vi "Text control 2 v5.4_pump-specific.vi"() -> ()   [LabVIEW 2016]
panel:
  in  "Tab Control":enum32{"Main", "Other parameters"}(tab)
  out "Line running":i32
  out "Total lines":i32
  out "Path":path=path "C:/users/rlp38/09Apr2009LTtesting/test2.txt"
  out "I vs Vg":cluster{"Y data in":dbl[], "X data in":dbl[]}[](graph)
  out "Is max":dbl format="%.2e"
  out "Id max":dbl format="%.2e"
  out "Ig max":dbl format="%.2e"
  out "Imax vs time":cluster{"Y data in":dbl[], "X data in":dbl[]}[](graph)
  out "Imin vs time":cluster{"Y data in":dbl[], "X data in":dbl[]}[](graph)
  out "I vs Vd":cluster{"Y data in":dbl[], "X data in":dbl[]}[](graph)
  in  "Script":string="#-------------------------------------------------------\n# SPM pump cleaning script\n#\n# Version 0.5\n# Author: Dimitrios Simatos\n# Last updated: 2018-01-05\n#-------------------------------------------------------\n# Description\n#\n# This script is designed to run the cleaning sequence of the SPM OEM pump.\n# This script needs to be run 4 times!\n#-------------------------------------------------------\n# Changes\n#\n# Placed initialization and hard stop commands in the beginning.\n#-------------------------------------------------------\n# Important points\n#\n# Never leave any liquid in the pump to dry after the experiments. If they dry, the residue may block the valve.\n# Always run the cleaning cycle after the experiments.\n# Use clockwise rotation when going up in valve port numbers and vice versa.\n#-------------------------------------------------------\n# Things to do before running the script\n#\n# Set time units to minutes.\n# Set filenames.\n# Replace the tubing, if necessary.\n#-------------------------------------------------------\n# Port connections\n#\n# Port 1: Waste\n# Port 2: Waste\n# Port 3: Various cleaning liquids\n# Port 4: Waste\n# Port 5: Waste\n# Port 6: Waste\n#\n# Between each of the 4 runs, the settings of Port 3 will change, according to the cleaning protocol.\n# The settings for Port 3 are:\n# 1st run: 1% v/v solution of sodium hypochlorite in ultrapure water\n# 2nd run: 0.1% w/v solution of sodium dodecyl sulfate in ultrapure water\n# 3rd run: Ultrapure water\n# 4th run: Waste (in air, not immersed in liquid)\n#-------------------------------------------------------\n# Cleaning protocol for the SPM OEM pump (from the manual)\n#\n# A cleaning procedure should be performed at the end of each day or in between two different experiments.\n# An effective cleaning can be performed in the following manner:\n# • Bleach solution to kill microorganisms\n# 1. Prepare a solution of 1% chlorine bleach and deionized water\n#    NOTE: Prepare a 1% v/v solution of sodium hypochlorite in deionized water\n# 2. Prepare a reservoir and place 1 tubing in the bleach solution and 5 tubings in a waste recipient\n# 3. Pick up the bleach solution through 1 port to entirely fill the syringe\n# 4. Sequentially output the syringe content through the remaining ports and throw it to the waste\n# 5. Repeat operation at least 2 times\n# • Detergent solution to remove debris\n# 1. Prepare a solution of 0.1% detergent and deionized water\n#    NOTE: Prepare a 0.1% w/v solution of sodium dodecyl sulfate in deionized water\n# 2. Move the tubing from the bleach solution reservoir and place it into a reservoir of detergent solution\n# 3. Pick up the detergent solution through 1 port to entirely fill the syringe\n# 4. Sequentially output the detergent solution through the remaining ports into the waste recipient\n# 5. Repeat operation at least 2 times\n# • Rinsing water to prepare the pump for your next experiment\n# 1. Move the tubing from the detergent solution reservoir and place it into a reservoir of deionized water\n# 2. Pick up the rinsing solution through 1 port to entirely fill the syringe\n# 3. Sequentially output the rinse water through the remaining ports into the waste recipient\n# 4. Repeat operation at least 2 times\n# • Replace the tubing, if necessary\n#-------------------------------------------------------\n# Pumping cycles and execution time\n#\n# Execution time for a single cycle: 6 x (1 min + 10 sec) = 7 minutes\n# Total execution time: 4 x 7 = 28 minutes\n# Since the script has to run 4 times, the cleaning lasts for: 4 x 28 = 112 minutes\n# Air must be the last to be pumped through the valve, to remove all liquids.\n# There are 4 pumping cycles. Each one draws a different liquid through port 3 and pumps it sequentially through ports 1,2,4,5,6.\n# During the sequential pumping, each port receives 200 ml of liquid (20% of the total syringe volume = 600 \"plunger units\")\n# The device must be disconnected from the port during the cleaning procedure.\n# All cycles are similar, except cycle 1 has the initialization command uncommented and the first report valve command commented.\n#-------------------------------------------------------\n# Volume of liquid needed\n#\n# Volume of liquid needed per cycle: 1 ml\n# Total volume of liquid needed per script run: 4 x 1 = 4 ml\n# Since the script has to run 4 times, the first 3 with different liquids, I need:\n# 4 ml of 1% v/v solution of sodium hypochlorite in ultrapure water\n# 4 ml of 0.1% w/v solution of sodium dodecyl sulfate in ultrapure water\n# 4 ml of ultrapure water\n#-------------------------------------------------------\n# Parameters\n#\n# Syringe size: 1 ml\n# Step resolution N = 0.01 mm\n# Drawing flow V = 300 pulses/second (6000 ul/min)\n# Pumping flow V = 300 pulses/second (6000 ul/min)\n#-------------------------------------------------------\n# Pump initialization\npump /1T #hard stop pump\npump /1ZR #initialize pump\n#-------------------------------------------------------\n# Cycle 1\n# Fill the syringe\npump /1Q #query pump\npump /1? #report absolute plunger position\n#pump /1?6 #report valve position\nwait-min 1 #wait 1 minute\npump /1N0R #set step resolution: 0.01 mm\npump /1Q #query pump\npump /1? #report absolute plunger position (the plunger should be at 0)\npump /1?6 #report valve position\nwait 1000 #wait 1 second\npump /1V300R #choose speed: 300 steps/s (6000 ul/min)\npump /1Q #query pump\nwait 1000 #wait 1 second\npump /1I3R #go to port 3, clockwise rotation\npump /1Q #query pump\npump /1?6 #report valve position\nwait 1000 #wait 1 second\npump /1A3000R #go to absolute position 3000 (= draw 1 ml)\nwait 30000 #wait 30 seconds\npump /1Q #query pump\npump /1? #report absolute plunger position (the plunger should have finished moving)\n#pump /1?6 #report valve position\n# The sequential pumping begins\n# Port 1\npump /1O1R #switch to port 1, counterclockwise rotation\npump /1Q #query pump\npump /1?6 #report valve position\npump /1A2400R #go to absolute position 2400 (= pump 200 ul)\npump /1Q #query pump\npump /1? #report absolute plunger position (the plunger should be moving to 0)\nwait-min 1 #wait 1 minute\npump /1? #report absolute plunger position (the plunger should have finished moving)\n# Port 2\npump /1I2R #switch to port 2, clockwise rotation\npump /1Q #query pump\npump /1?6 #report valve position\npump /1A1800R #go to absolute position 1800 (= pump 200 ul)\npump /1Q #query pump\npump /1? #report absolute plunger position (the plunger should be moving to 0)\nwait-min 1 #wait 1 minute\npump /1? #report absolute plunger position (the plunger should have finished moving)\n# Port 4\npump /1I4R #switch to port 4, clockwise rotation\npump /1Q #query pump\npump /1?6 #report valve position\npump /1A1200R #go to absolute position 1200 (= pump 200 ul)\npump /1Q #query pump\npump /1? #report absolute plunger position (the plunger should be moving to 0)\nwait-min 1 #wait 1 minute\npump /1? #report absolute plunger position (the plunger should have finished moving)\n# Port 5\npump /1I5R #switch to port 5, clockwise rotation\npump /1Q #query pump\npump /1?6 #report valve position\npump /1A600R #go to absolute position 600 (= pump 200 ul)\npump /1Q #query pump\npump /1? #report absolute plunger position (the plunger should be moving to 0)\nwait-min 1 #wait 1 minute\npump /1? #report absolute plunger position (the plunger should have finished moving)\n# Port 6\npump /1I6R #switch to port 6, clockwise rotation\npump /1Q #query pump\npump /1?6 #report valve position\npump /1A0R #go to absolute position 0 (= pump 200 ul)\npump /1Q #query pump\npump /1? #report absolute plunger position (the plunger should be moving to 0)\nwait-min 1 #wait 1 minute\npump /1? #report absolute plunger position (the plunger should have finished moving)\n#-------------------------------------------------------\n# Cycle 2\n# Fill the syringe\n#pump /1ZR #initialize pump\npump /1Q #query pump\npump /1? #report absolute plunger position\npump /1?6 #report valve position\nwait-min 1 #wait 1 minute\npump /1N0R #set step resolution: 0.01 mm\npump /1Q #query pump\npump /1? #report absolute plunger position (the plunger should be at 0)\npump /1?6 #report valve position\nwait 1000 #wait 1 second\npump /1V300R #choose speed: 300 steps/s (6000 ul/min)\npump /1Q #query pump\nwait 1000 #wait 1 second\npump /1O3R #go to port 3, counterclockwise rotation\npump /1Q #query pump\npump /1?6 #report valve position\nwait 1000 #wait 1 second\npump /1A3000R #go to absolute position 3000 (= draw 1 ml)\nwait 30000 #wait 30 seconds\npump /1Q #query pump\npump /1? #report absolute plunger position (the plunger should have finished moving)\n#pump /1?6 #report valve position\n# The sequential pumping begins\n# Port 1\npump /1O1R #switch to port 1, counterclockwise rotation\npump /1Q #query pump\npump /1?6 #report valve position\npump /1A2400R #go to absolute position 2400 (= pump 200 ul)\npump /1Q #query pump\npump /1? #report absolute plunger position (the plunger should be moving to 0)\nwait-min 1 #wait 1 minute\npump /1? #report absolute plunger position (the plunger should have finished moving)\n# Port 2\npump /1I2R #switch to port 2, clockwise rotation\npump /1Q #query pump\npump /1?6 #report valve position\npump /1A1800R #go to absolute position 1800 (= pump 200 ul)\npump /1Q #query pump\npump /1? #report absolute plunger position (the plunger should be moving to 0)\nwait-min 1 #wait 1 minute\npump /1? #report absolute plunger position (the plunger should have finished moving)\n# Port 4\npump /1I4R #switch to port 4, clockwise rotation\npump /1Q #query pump\npump /1?6 #report valve position\npump /1A1200R #go to absolute position 1200 (= pump 200 ul)\npump /1Q #query pump\npump /1? #report absolute plunger position (the plunger should be moving to 0)\nwait-min 1 #wait 1 minute\npump /1? #report absolute plunger position (the plunger should have finished moving)\n# Port 5\npump /1I5R #switch to port 5, clockwise rotation\npump /1Q #query pump\npump /1?6 #report valve position\npump /1A600R #go to absolute position 600 (= pump 200 ul)\npump /1Q #query pump\npump /1? #report absolute plunger position (the plunger should be moving to 0)\nwait-min 1 #wait 1 minute\npump /1? #report absolute plunger position (the plunger should have finished moving)\n# Port 6\npump /1I6R #switch to port 6, clockwise rotation\npump /1Q #query pump\npump /1?6 #report valve position\npump /1A0R #go to absolute position 0 (= pump 200 ul)\npump /1Q #query pump\npump /1? #report absolute plunger position (the plunger should be moving to 0)\nwait-min 1 #wait 1 minute\npump /1? #report absolute plunger position (the plunger should have finished moving)\n#-------------------------------------------------------\n# Cycle 3\n# Fill the syringe\n#pump /1ZR #initialize pump\npump /1Q #query pump\npump /1? #report absolute plunger position\npump /1?6 #report valve position\nwait-min 1 #wait 1 minute\npump /1N0R #set step resolution: 0.01 mm\npump /1Q #query pump\npump /1? #report absolute plunger position (the plunger should be at 0)\npump /1?6 #report valve position\nwait 1000 #wait 1 second\npump /1V300R #choose speed: 300 steps/s (6000 ul/min)\npump /1Q #query pump\nwait 1000 #wait 1 second\npump /1O3R #go to port 3, counterclockwise rotation\npump /1Q #query pump\npump /1?6 #report valve position\nwait 1000 #wait 1 second\npump /1A3000R #go to absolute position 3000 (= draw 1 ml)\nwait 30000 #wait 30 seconds\npump /1Q #query pump\npump /1? #report absolute plunger position (the plunger should have finished moving)\n#pump /1?6 #report valve position\n# The sequential pumping begins\n# Port 1\npump /1O1R #switch to port 1, counterclockwise rotation\npump /1Q #query pump\npump /1?6 #report valve position\npump /1A2400R #go to absolute position 2400 (= pump 200 ul)\npump /1Q #query pump\npump /1? #report absolute plunger position (the plunger should be moving to 0)\nwait-min 1 #wait 1 minute\npump /1? #report absolute plunger position (the plunger should have finished moving)\n# Port 2\npump /1I2R #switch to port 2, clockwise rotation\npump /1Q #query pump\npump /1?6 #report valve position\npump /1A1800R #go to absolute position 1800 (= pump 200 ul)\npump /1Q #query pump\npump /1? #report absolute plunger position (the plunger should be moving to 0)\nwait-min 1 #wait 1 minute\npump /1? #report absolute plunger position (the plunger should have finished moving)\n# Port 4\npump /1I4R #switch to port 4, clockwise rotation\npump /1Q #query pump\npump /1?6 #report valve position\npump /1A1200R #go to absolute position 1200 (= pump 200 ul)\npump /1Q #query pump\npump /1? #report absolute plunger position (the plunger should be moving to 0)\nwait-min 1 #wait 1 minute\npump /1? #report absolute plunger position (the plunger should have finished moving)\n# Port 5\npump /1I5R #switch to port 5, clockwise rotation\npump /1Q #query pump\npump /1?6 #report valve position\npump /1A600R #go to absolute position 600 (= pump 200 ul)\npump /1Q #query pump\npump /1? #report absolute plunger position (the plunger should be moving to 0)\nwait-min 1 #wait 1 minute\npump /1? #report absolute plunger position (the plunger should have finished moving)\n# Port 6\npump /1I6R #switch to port 6, clockwise rotation\npump /1Q #query pump\npump /1?6 #report valve position\npump /1A0R #go to absolute position 0 (= pump 200 ul)\npump /1Q #query pump\npump /1? #report absolute plunger position (the plunger should be moving to 0)\nwait-min 1 #wait 1 minute\npump /1? #report absolute plunger position (the plunger should have finished moving)\n#-------------------------------------------------------\n# Cycle 4\n# Fill the syringe\n#pump /1ZR #initialize pump\npump /1Q #query pump\npump /1? #report absolute plunger position\npump /1?6 #report valve position\nwait-min 1 #wait 1 minute\npump /1N0R #set step resolution: 0.01 mm\npump /1Q #query pump\npump /1? #report absolute plunger position (the plunger should be at 0)\npump /1?6 #report valve position\nwait 1000 #wait 1 second\npump /1V300R #choose speed: 300 steps/s (6000 ul/min)\npump /1Q #query pump\nwait 1000 #wait 1 second\npump /1O3R #go to port 3, counterclockwise rotation\npump /1Q #query pump\npump /1?6 #report valve position\nwait 1000 #wait 1 second\npump /1A3000R #go to absolute position 3000 (= draw 1 ml)\nwait 30000 #wait 30 seconds\npump /1Q #query pump\npump /1? #report absolute plunger position (the plunger should have finished moving)\n#pump /1?6 #report valve position\n# The sequential pumping begins\n# Port 1\npump /1O1R #switch to port 1, counterclockwise rotation\npump /1Q #query pump\npump /1?6 #report valve position\npump /1A2400R #go to absolute position 2400 (= pump 200 ul)\npump /1Q #query pump\npump /1? #report absolute plunger position (the plunger should be moving to 0)\nwait-min 1 #wait 1 minute\npump /1? #report absolute plunger position (the plunger should have finished moving)\n# Port 2\npump /1I2R #switch to port 2, clockwise rotation\npump /1Q #query pump\npump /1?6 #report valve position\npump /1A1800R #go to absolute position 1800 (= pump 200 ul)\npump /1Q #query pump\npump /1? #report absolute plunger position (the plunger should be moving to 0)\nwait-min 1 #wait 1 minute\npump /1? #report absolute plunger position (the plunger should have finished moving)\n# Port 4\npump /1I4R #switch to port 4, clockwise rotation\npump /1Q #query pump\npump /1?6 #report valve position\npump /1A1200R #go to absolute position 1200 (= pump 200 ul)\npump /1Q #query pump\npump /1? #report absolute plunger position (the plunger should be moving to 0)\nwait-min 1 #wait 1 minute\npump /1? #report absolute plunger position (the plunger should have finished moving)\n# Port 5\npump /1I5R #switch to port 5, clockwise rotation\npump /1Q #query pump\npump /1?6 #report valve position\npump /1A600R #go to absolute position 600 (= pump 200 ul)\npump /1Q #query pump\npump /1? #report absolute plunger position (the plunger should be moving to 0)\nwait-min 1 #wait 1 minute\npump /1? #report absolute plunger position (the plunger should have finished moving)\n# Port 6\npump /1I6R #switch to port 6, clockwise rotation\npump /1Q #query pump\npump /1?6 #report valve position\npump /1A0R #go to absolute position 0 (= pump 200 ul)\npump /1Q #query pump\npump /1? #report absolute plunger position (the plunger should be moving to 0)\nwait-min 1 #wait 1 minute\npump /1? #report absolute plunger position (the plunger should have finished moving)\n#-------------------------------------------------------"
  out "Command running:":string
  out "Serial port data":string
  out "Elapsed Time":dbl caption="Elapsed Time (s)"
  in  "Units":u16(ring)=1 items=["Seconds", "Minutes", "Hours"]
  in  "Time Offset":dbl caption="Set Start Time (s)"
  in  "Reset":bool
  in  "Auto Reset":bool
  in  "integration time":u32(slide) max=2 step=1 scale=0.0..2.0
  in  "Interrupt run":bool
  out "Absolute plunger position vs time":cluster{"Y data in":dbl[], "X data in":dbl[]}[](graph)
  out "Valve position vs time":cluster{"Y data in":dbl[], "X data in":dbl[]}[](graph)
  in  "Halt pump":bool
  in  "Hard stop pump":bool
  out "Is on":dbl format="%.2e"
  out "Id on":dbl format="%.2e"
  out "Ig on":dbl format="%.2e"
  out "Ion vs time":cluster{"Y data in":dbl[], "X data in":dbl[]}[](graph)
  out "Ioff vs time":cluster{"Y data in":dbl[], "X data in":dbl[]}[](graph)
  out "Ig min":dbl format="%.2e"
  out "Id min":dbl format="%.2e"
  out "Is min":dbl format="%.2e"
  out "Is off":dbl format="%.2e"
  out "Id off":dbl format="%.2e"
  out "Ig off":dbl format="%.2e"
  in  "Gate Range\nmode":u16(ring) items=["Auto", "Limited", "Fixed"]
  in  "Gate Range":u8(slide)=6 max=11 scale=0.0..11.0
  in  "Source/Drain\nRange mode":u16(ring) items=["Auto", "Limited", "Fixed"]
  in  "Source/Drain Range":u8(slide)=6 max=11 scale=0.0..11.0
  in  "Panel Controls":T1={"Emergency Stop"=refnum, "TransGraph Max"=1e-05, "Text/Graph (text=false)"=TRUE} {"TransGraph Max" format="%.2e"}
  in  "Panel Controls 2":T2={"Emergency Stop"=refnum, "TransGraph Max"=1e-05, "Text/Graph (text=false)"=TRUE, "TransGraph Min"=1e-11} {"TransGraph Min" format="%.2e"; "TransGraph Max" format="%.2e"}
  in  "SMU4":cluster{"on/off":bool, "Voltage":dbl} {"Voltage" min=-100.0 max=100.0 format="%.2f"}
  in  "Full Reset":bool
  in  "Standby":T3
  out "error out":errorcluster
  in  "Delay before read (ms)":u32=1000
  in  "byte count":u32=64
  in  "Serial End Mode for Reads":u16(ring)=2 items=["None", "LastBit", "TermChar"]
  in  "Timeout (ms)":u32=10000
  in  "Enable Termination\nChar (T)":bool=TRUE
  in  "Termination char\n(0xA = '\\n' = LF)\n(0xD = '\\r' = CR)":u8=13 format="%.0x"
  in  "flow control":u16(ring) items=["None"=0, "XON/XOFF"=1, "RTS/CTS"=2, "DTR/DSR"=4]
  in  "stop bits":u16(ring)=10 items=["1.0"=10, "1.5"=15, "2.0"=20]
  in  "parity":u16(ring) items=["None", "Odd", "Even", "Mark", "Space"]
  in  "data bits":u16=8 min=5 max=8 step=1
  in  "VISA resource name":refnum<visa-resource-name>="COM6"
  in  "baud rate":u32=9600
  in  "Drain: Compliance":dbl=0.001 format="%.8f"
  in  "Gate: Compliance":dbl=0.001 format="%.8f"
  in  "hold time /s":dbl format="%.2f"
  in  "delay time /s":dbl format="%.2f"
  in  "Integration time (short)":dbl=0.0019 min=8e-05 max=0.0019 step=8e-05 format="%^.0e"
  in  "Integration time (long)":dbl=0.32 min=0.04 max=2.0 step=0.02 format="%.2f"
  in  "Step delay /s":dbl format="%.2f"
  in  "Filename (variable part)":string="step_1_up-H2O_initial_"
  in  "Suffix (script)":string="script.txt"
  in  "Gate":T4={"Gate Start"=0.0, "Gate Stop"=2.0, "Gate Step (linear only)"=1.0, "Gate Compliance"=0.0001, "Gate PComp"=0.0, "Range mode"=0, "Range"=6} {"Range" max=11 scale=0.0..11.0; "Range mode" items=["Auto", "Limited", "Fixed"]; "Gate PComp" format="%^.2e"; "Gate Compliance" format="%^.2e"; "Gate Step (linear only)" format="%^.4e"; "Gate Stop" format="%^.4e"; "Gate Start" format="%^.4e"}
  in  "Drain 2":T5={"Drain Start"=0.0, "Drain Stop"=2.0, "Drain Compliance"=0.0001, "Drain Step"=1.0, "Drain PComp"=0.0, "Range mode"=0, "Range"=6} {"Range" max=11 scale=0.0..11.0; "Range mode" items=["Auto", "Limited", "Fixed"]; "Drain PComp" format="%^.2e"; "Drain Step" format="%^.4e"; "Drain Compliance" format="%^.2e"; "Drain Stop" format="%^.4e"; "Drain Start" format="%^.4e"}
  in  "Timings 2":T6={"integration time"=0, "Short/Long integration time"=0.00064, "hold time (sec)"=0.0, "delay time (sec)"=0.0, "Step Time (0 disables)"=0.0, "sweep method"=0, "Pulse period"=0.005, "Base voltage"=0.0, "Pulse width"=0.0005} {"Pulse width" min=0.0005 max=0.1 step=0.0001 format="%.4f"; "Base voltage" format="%^.4e"; "Pulse period" min=0.005 max=1.0 step=0.0001 format="%.4f"; "sweep method" items=["Continuous", "Pulsed"]; "Step Time (0 disables)" format="%.2f"; "delay time (sec)" format="%.4f"; "hold time (sec)" format="%.4f"; "Short/Long integration time" format="%^.0e"; "integration time" scale=0.0..2.0}
  # "Syntax:\nitime [s|m|l]\ngaterangemode [a|l|f]\ndrainrangemode [a|l|f]\npulsed [on|off] PulsePeriod(sec) PulseBaseVoltage PulseONWidth(sec)\nstandby [on l off]\nwait NumMilliseconds\nwait-min NumMinutes\n# texthere = comment\ntransfer [s|d] VgStart VgStop VgStep VdStart VdStop VdStep\noutput [s|d] VgStart VgStop VgStep VdStart VdStop VdStep\nsample Vg Vd NumSamples Time(s) SampleInterval(s)\nsamplei Idg NumSamples Time(s) SampleInterval(s) VDGcompliance\n100 samples is approximately 13 seconds with medium integration\n# if in doubt use SampleInterval(s) = 0.004\nstressV VG VD IGcompliance IDcompliance Duration(sec)\nstressI IDG VDGcompliance Duration(sec)\nvsu2pulse Bias Duration(s)\npulsedstressV [s|d] VEstop VgON VgOFF Period(s) PulseONwidth(s) Vd\nsample-fpp Vg Vd NumSamples Time\nresample-fpp Vg Vd\ntransfer-fpp [s|d] VgStart VgStop VgStep VdStart VdStop VdStep\noutput-fpp [s|d] VgStart VgStop VgStep VdStart VdStop VdStep\nserial SerialPortCommand\npump SerialPortCommand for the SPM pump\n\nSPM Pump Syntax (<x>: pump number, use 1 if only one pump):\nif the command syntax contains [R], then append the letter R to the command\n/<x>Q: query (a query command should follow each command)\n/<x>Z[R] or /<x>Y[R]: initialize pump\n/<x>N<n>[R] (<n>=0,1): <0> (<1>) microstep 0.01 mm (0.00125 mm) resolution\n/<x>I<n> (<n>=0-6): turn to port number n (clockwise)\n/<x>O<n> (<n>=0-6): turn to port number n (counterclockwise)\n/<x>X: Re-execute last command string\n/<x>G<n>[R] (<n>=0-60000): repeat command sequence (default: 0, 0=loop forever)\n/<x>g: Mark the start of a repeat sequence (max = 10)\n/<x>M<n>[R] (<n>=0-86400000): delay command execution by n milliseconds\n/<x>H: Halt; Pause the sequence after finishing the current move\n/<x>T: Hardstop; Interrupt the current move and suppress it from the sequence\n/<x>A<n>[R] (<n>=0-3000 with N=0, 0-24000 with N=1): absolute position\n/<x>P<n>[R] (<n>=0-3000 with N=0, 0-24000 with N=1): relative pickup\n/<x>D<n>[R] (<n>=0-3000 with N=0, 0-24000 with N=1): relative dispense\n/<x>V<n>[R] (<n>=1-1600 default: 150): set peak speed (pulses/sec)\nNOTE: The lowest speed limit is 1 pulse/sec, not 5, as the manual states.\n/<x>S<n>[R] (<n>=10-40 default: 22): set speed (NOT in pulses/sec, look in manual)\nNOTE: When controlled with absolute position, one does not need to pay special attention to the syringe that is mounted on the pump.\nWithdraw from lower stage (ports 3, 5), dispense from higher stage (ports 2, 4, 6).\nConnect Port 1 to waste."
  # "Time"
  # "1\n2\n3\n4\n5\n6\n7\n8\n9\n10\n11\n12\n13\n14\n15\n16\n17\n18\n19\n20"
  # "Serial port settings"
  # "Filename settings"
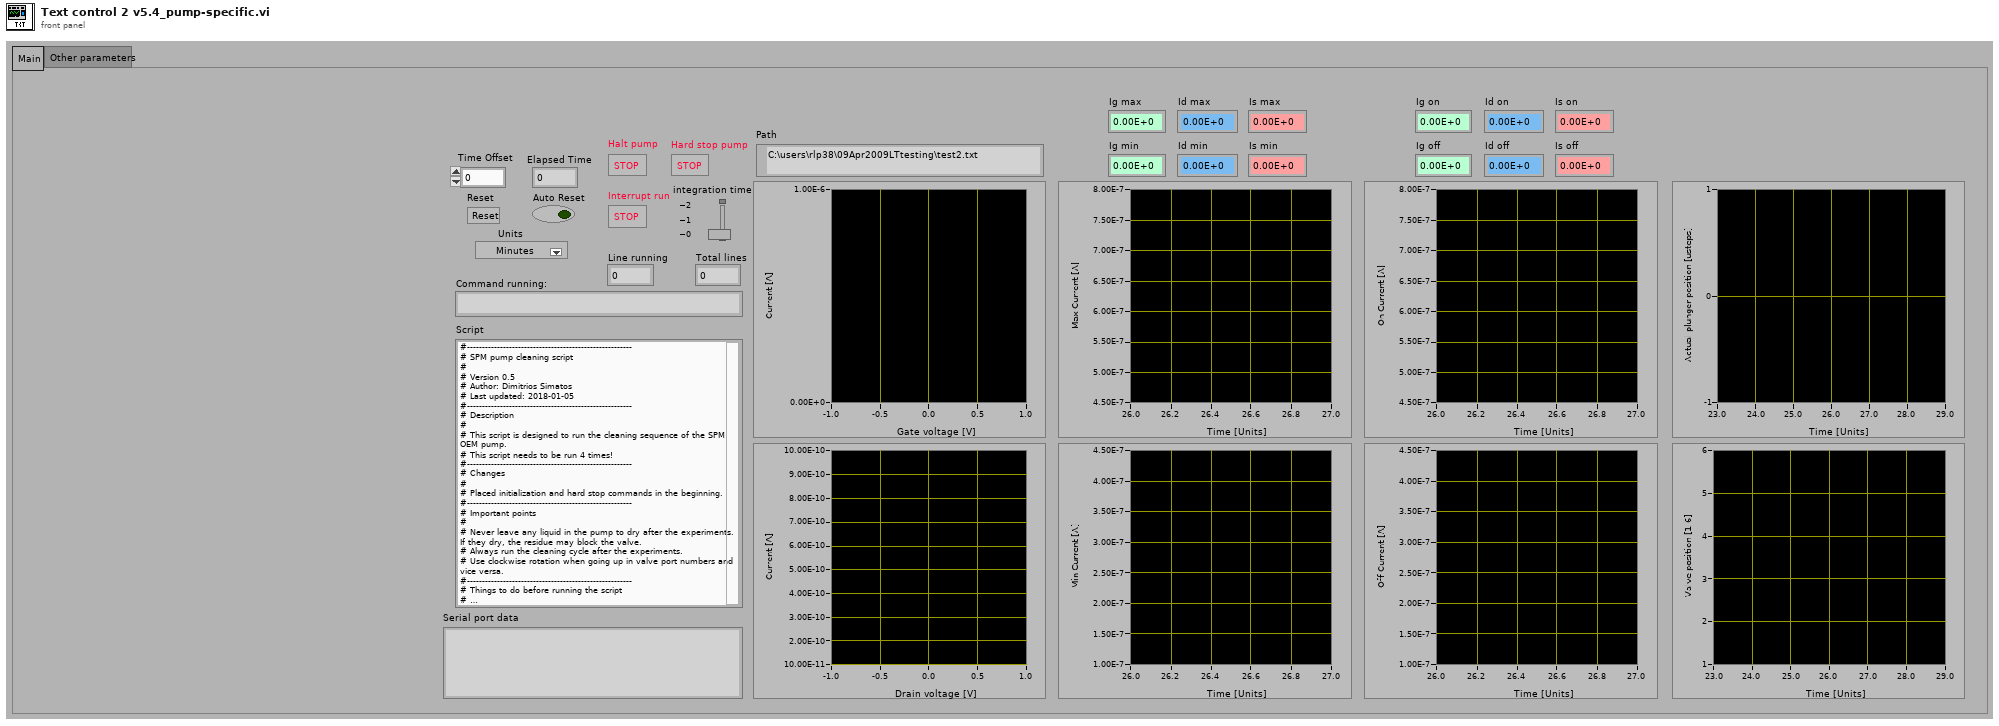
[diagram p1: front panel]
types:
  T1 = cluster{"Emergency Stop":refnum<vi>, "TransGraph Max":dbl, "Text/Graph (text=false)":bool}
  T2 = cluster{"Emergency Stop":refnum<vi>, "TransGraph Max":dbl, "Text/Graph (text=false)":bool, "TransGraph Min":dbl}
  T3 = cluster{"Gate Standby":bool, "Drain Standby":bool}
  T4 = cluster{"Gate Start":dbl, "Gate Stop":dbl, "Gate Step (linear only)":dbl, "Gate Compliance":dbl, "Gate PComp":dbl, "Range mode":u16, "Range":u8}
  T5 = cluster{"Drain Start":dbl, "Drain Stop":dbl, "Drain Compliance":dbl, "Drain Step":dbl, "Drain PComp":dbl, "Range mode":u16, "Range":u8}
  T6 = cluster{"integration time":u32, "Short/Long integration time":dbl, "hold time (sec)":dbl, "delay time (sec)":dbl, "Step Time (0 disables)":dbl, "sweep method":u16, "Pulse period":dbl, "Base voltage":dbl, "Pulse width":dbl}
  T7 = enum16{"open", "replace", "create", "open or create", "replace or create", "replace or create with confirmation"}
  T8 = cluster{"V2 Start":dbl, "V2 Step":dbl, "Number of points":i32}
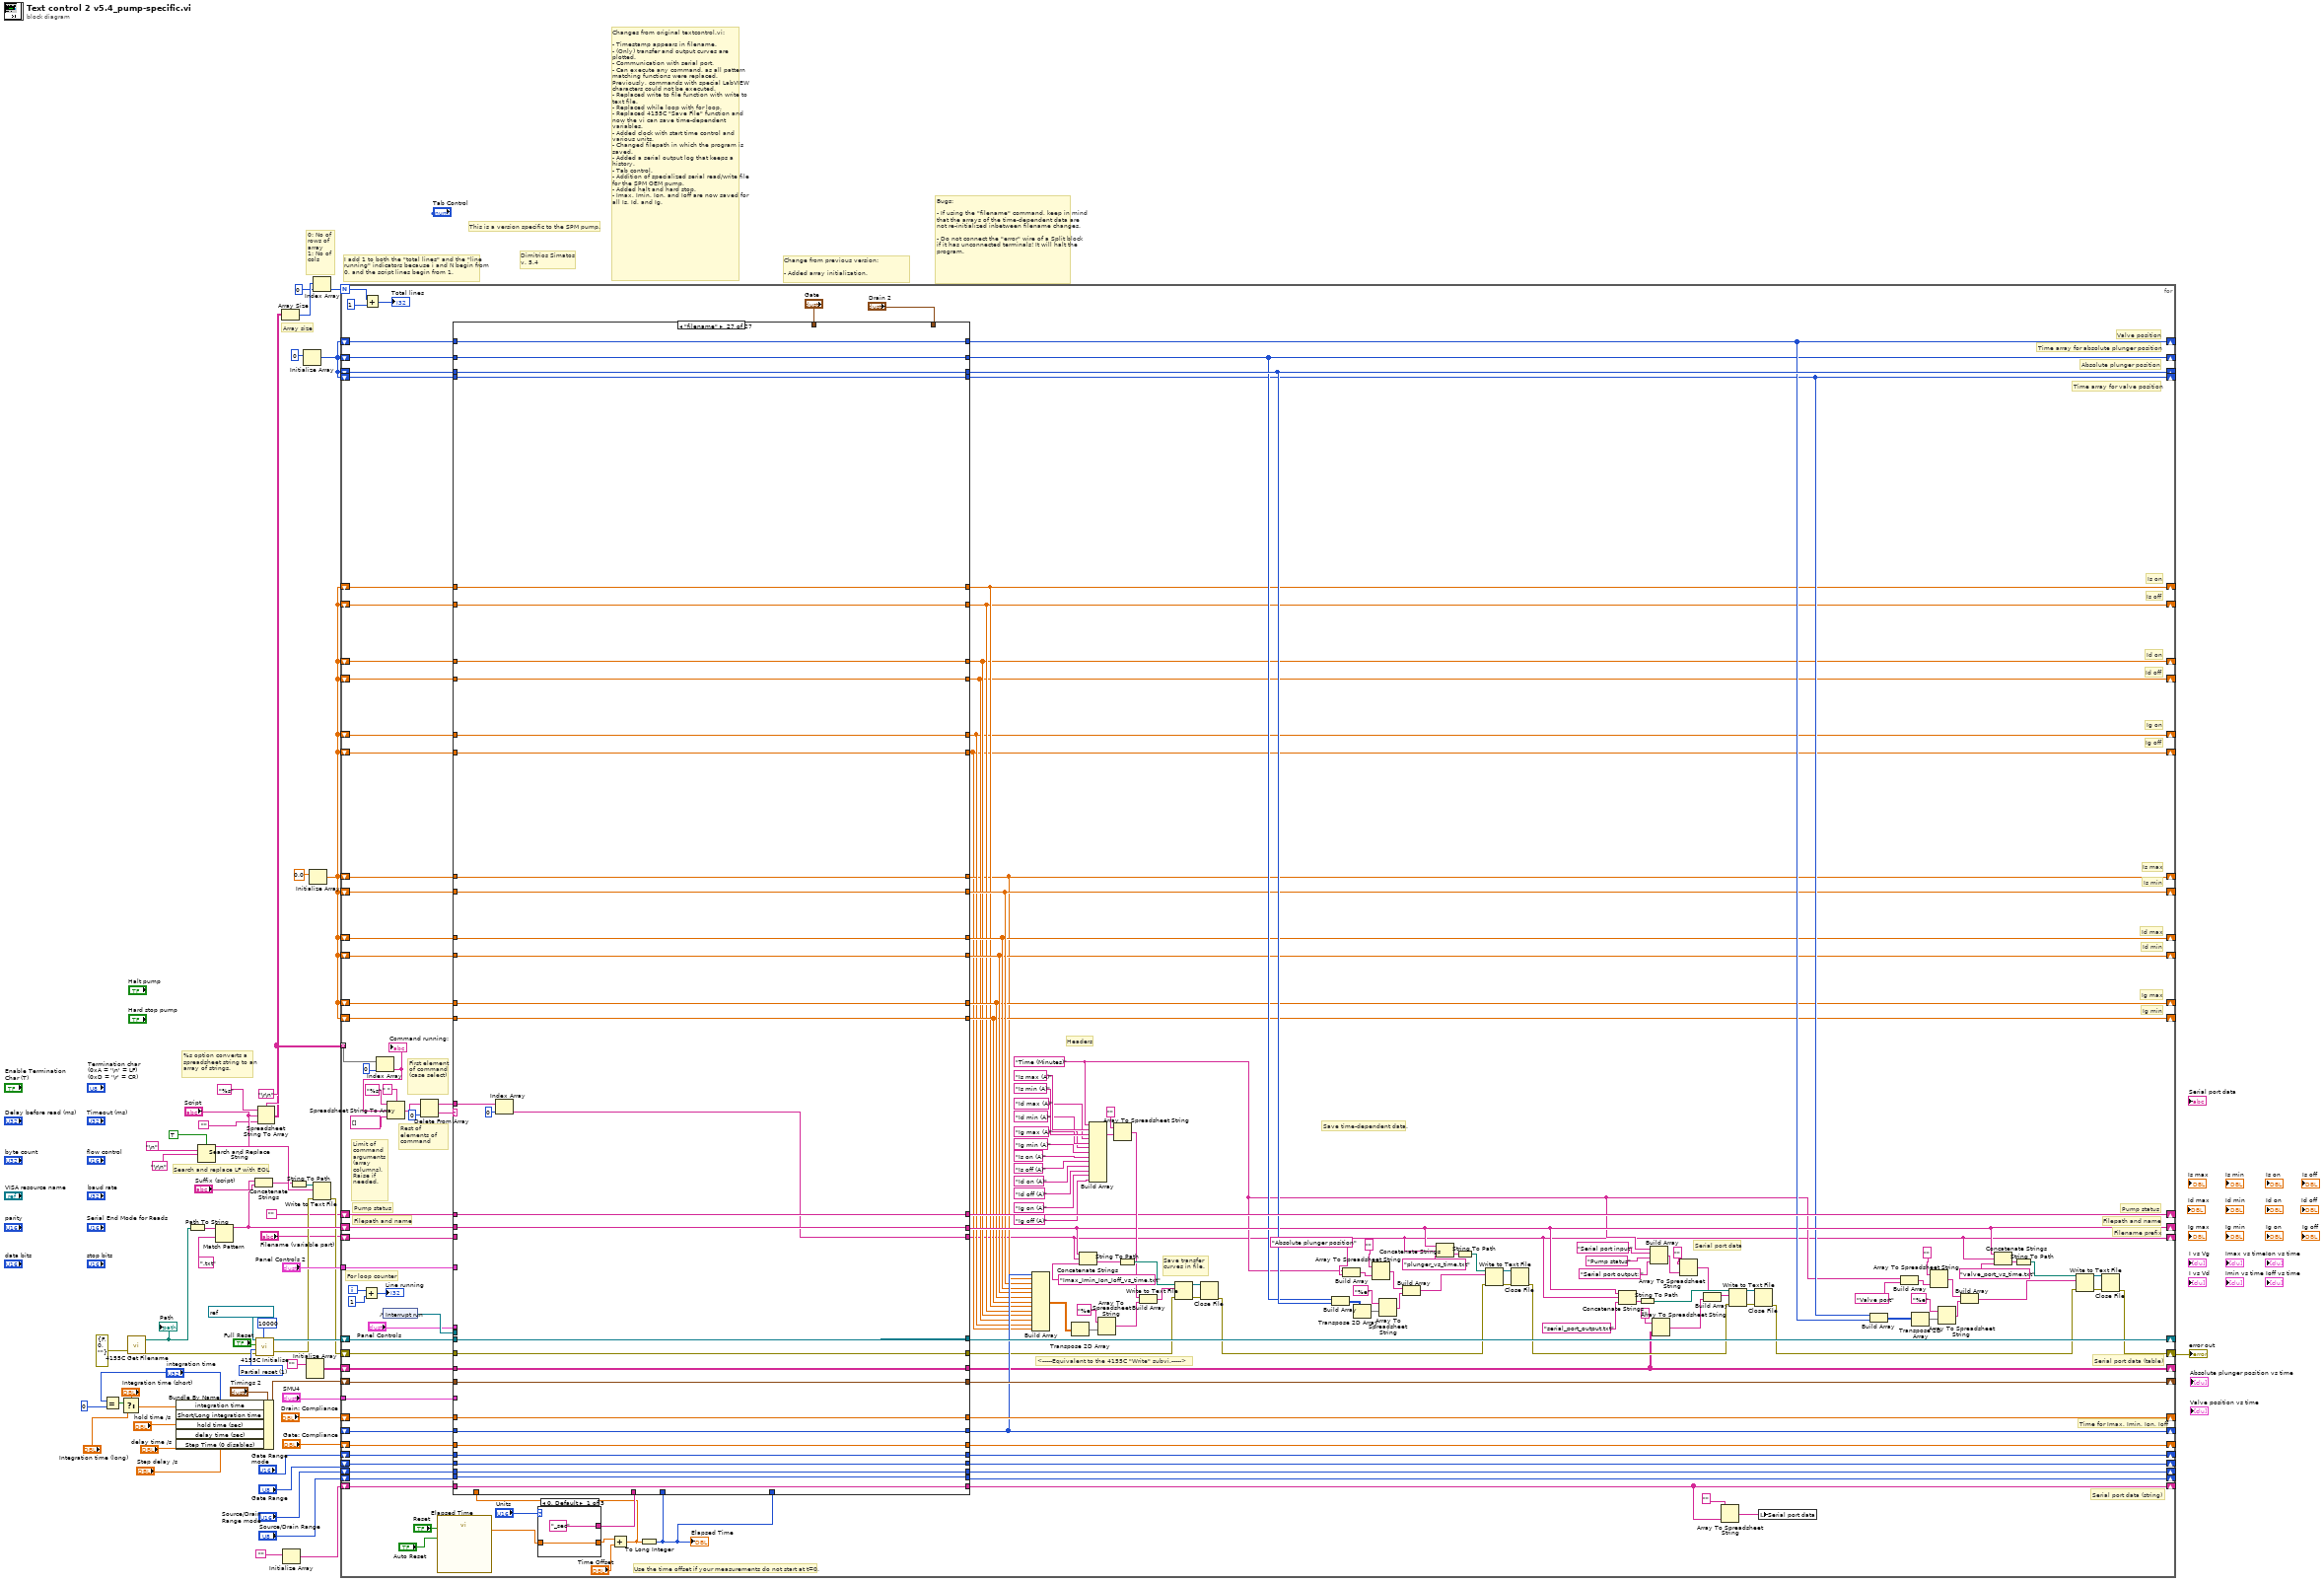
[diagram p0: block diagram]
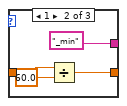
[diagram p2: hidden frame]
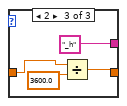
[diagram p3: hidden frame]
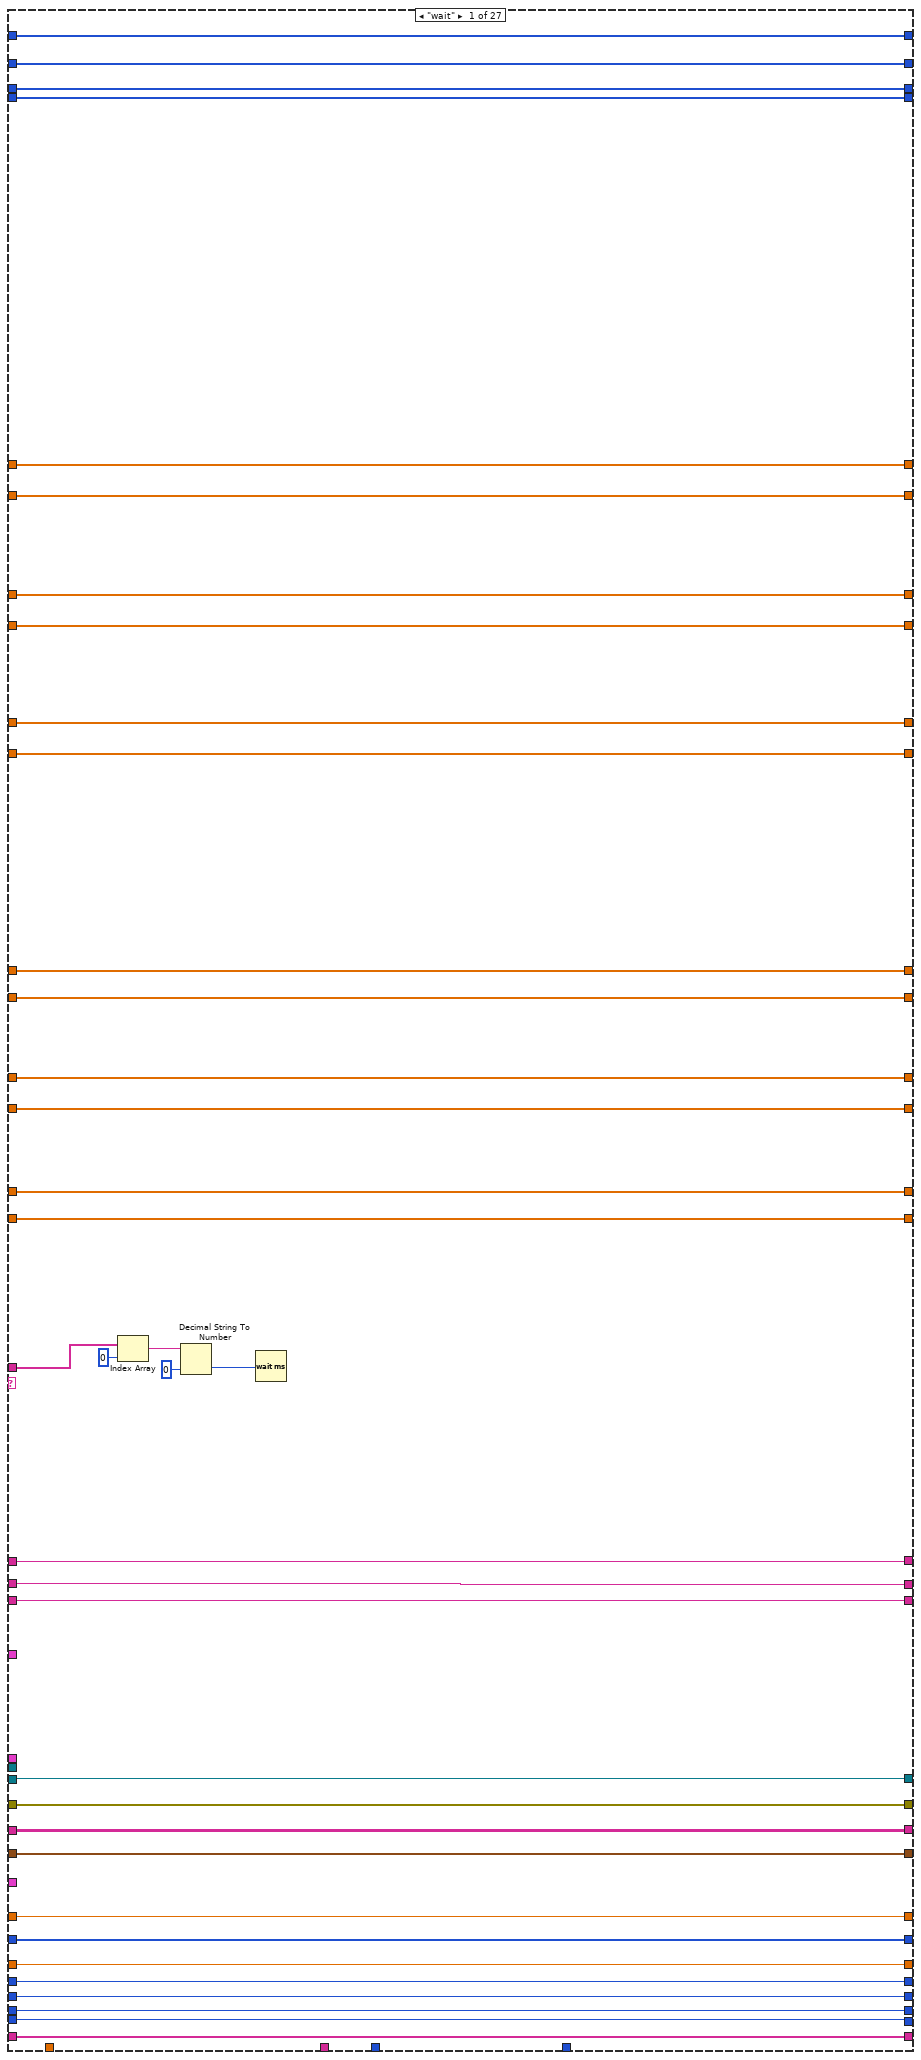
[diagram p4: hidden frame]
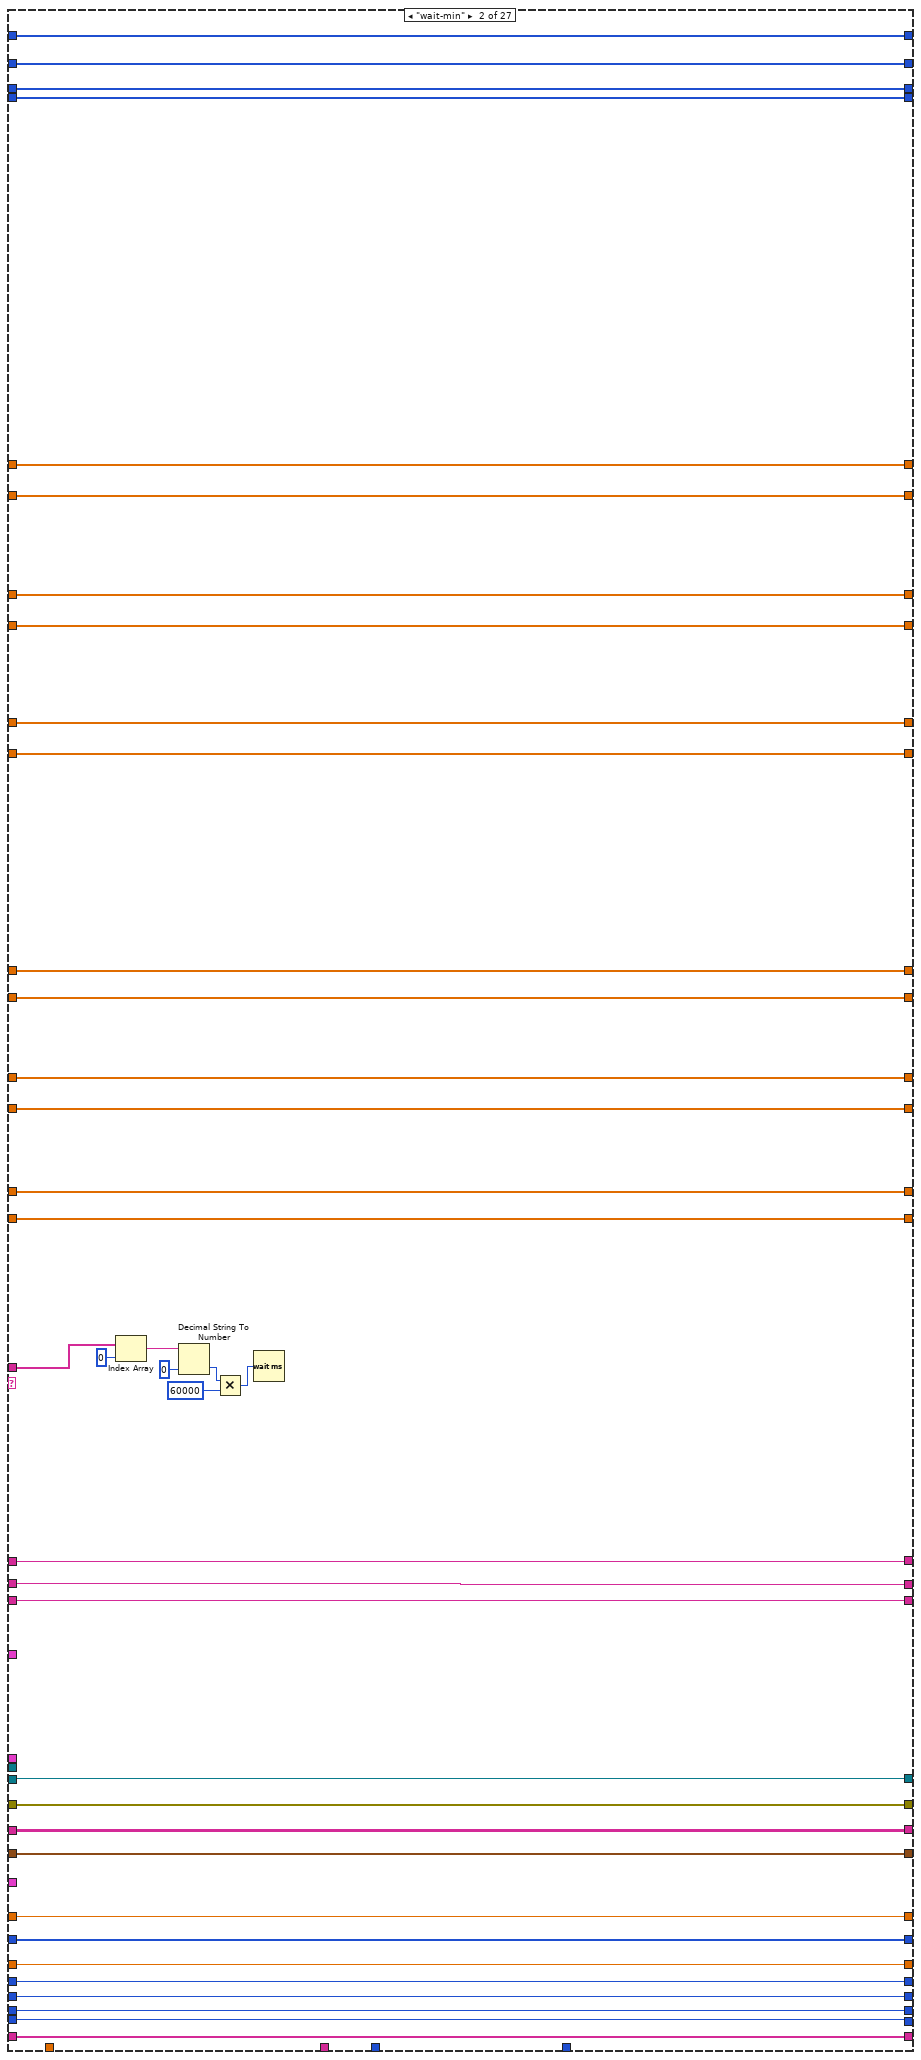
[diagram p5: hidden frame]
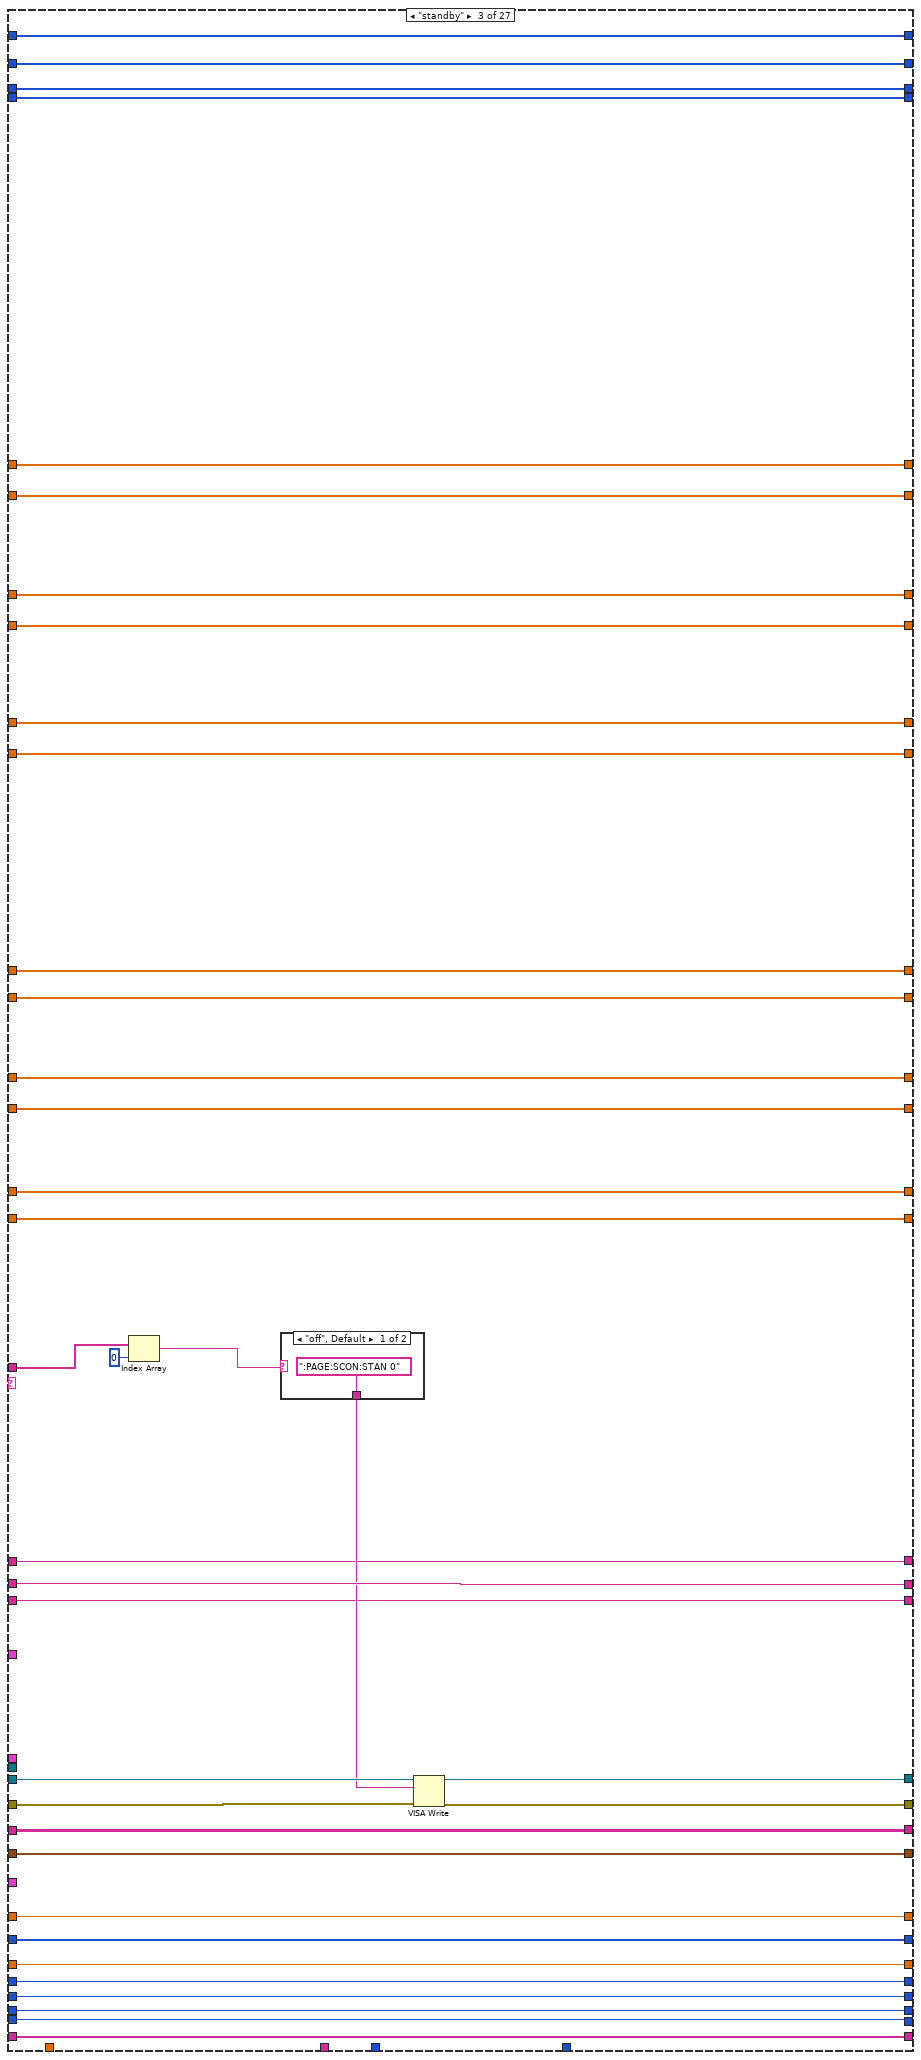
[diagram p6: hidden frame]
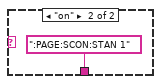
[diagram p7: hidden frame]
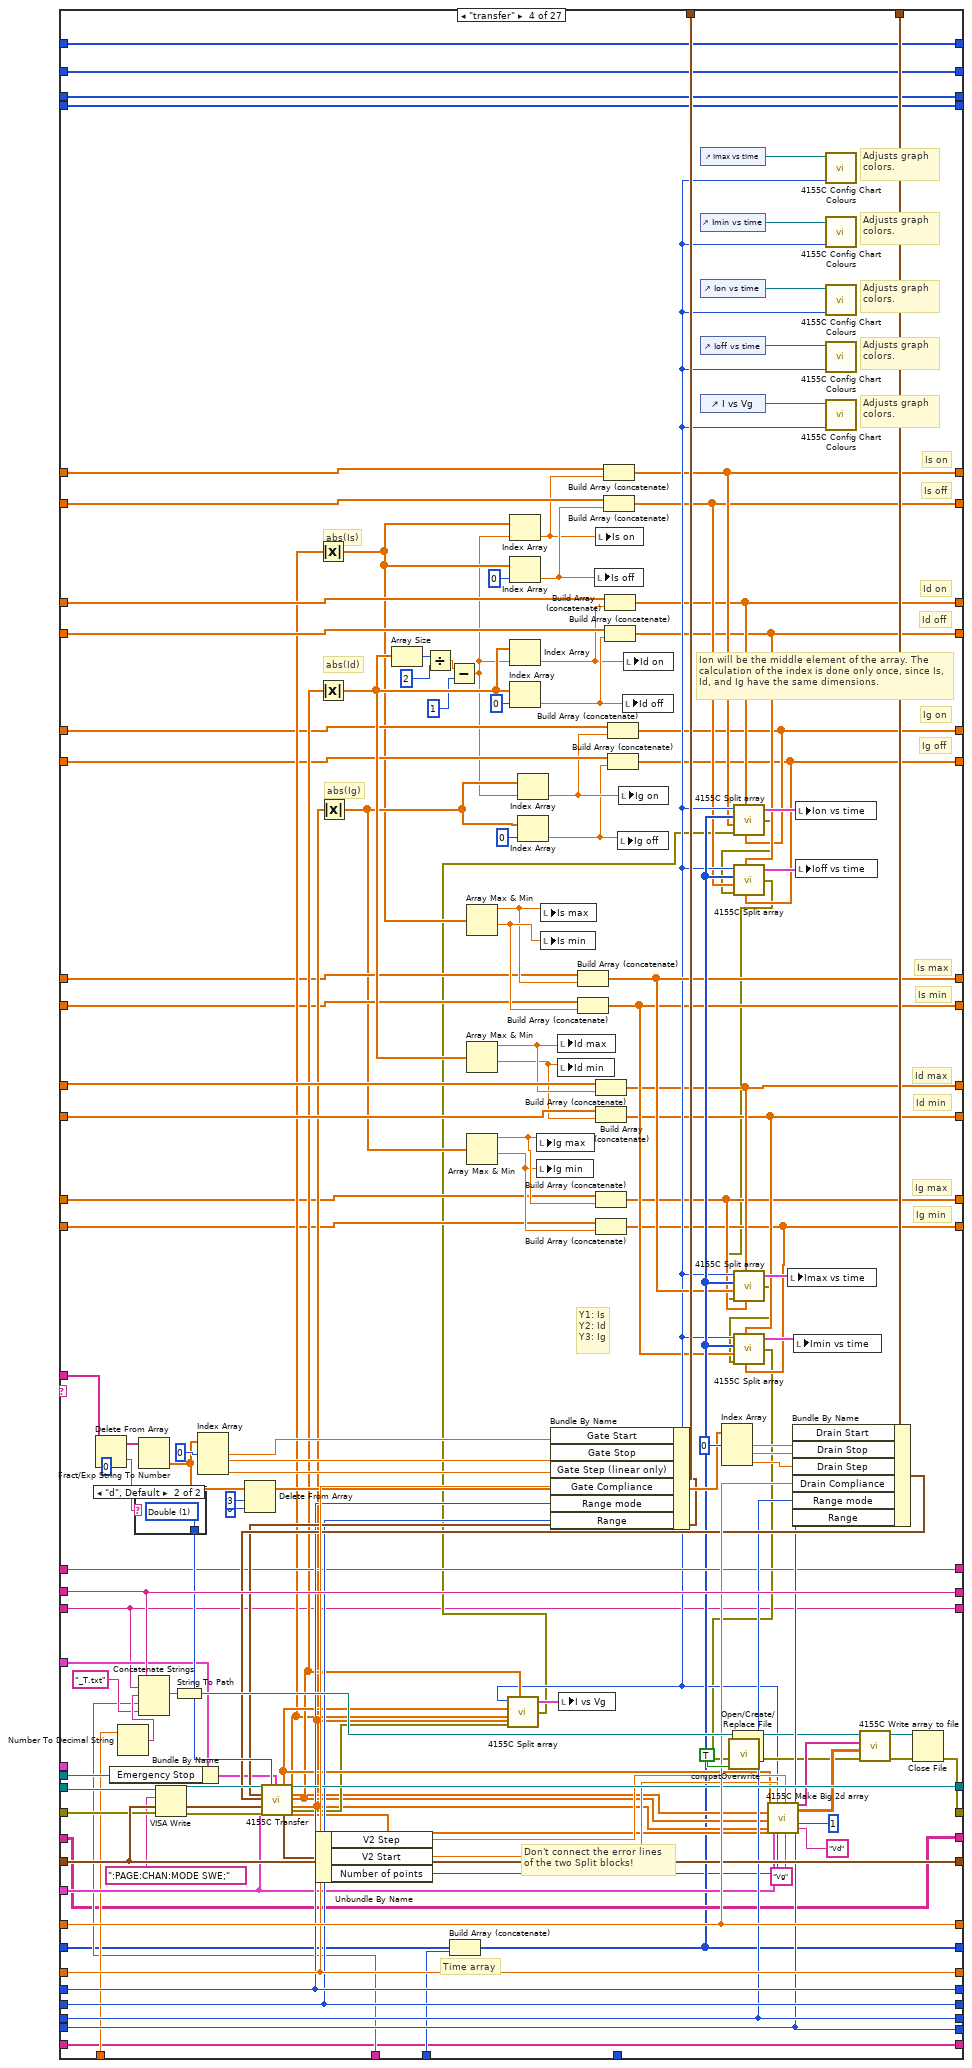
[diagram p8: hidden frame]
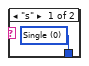
[diagram p9: hidden frame]
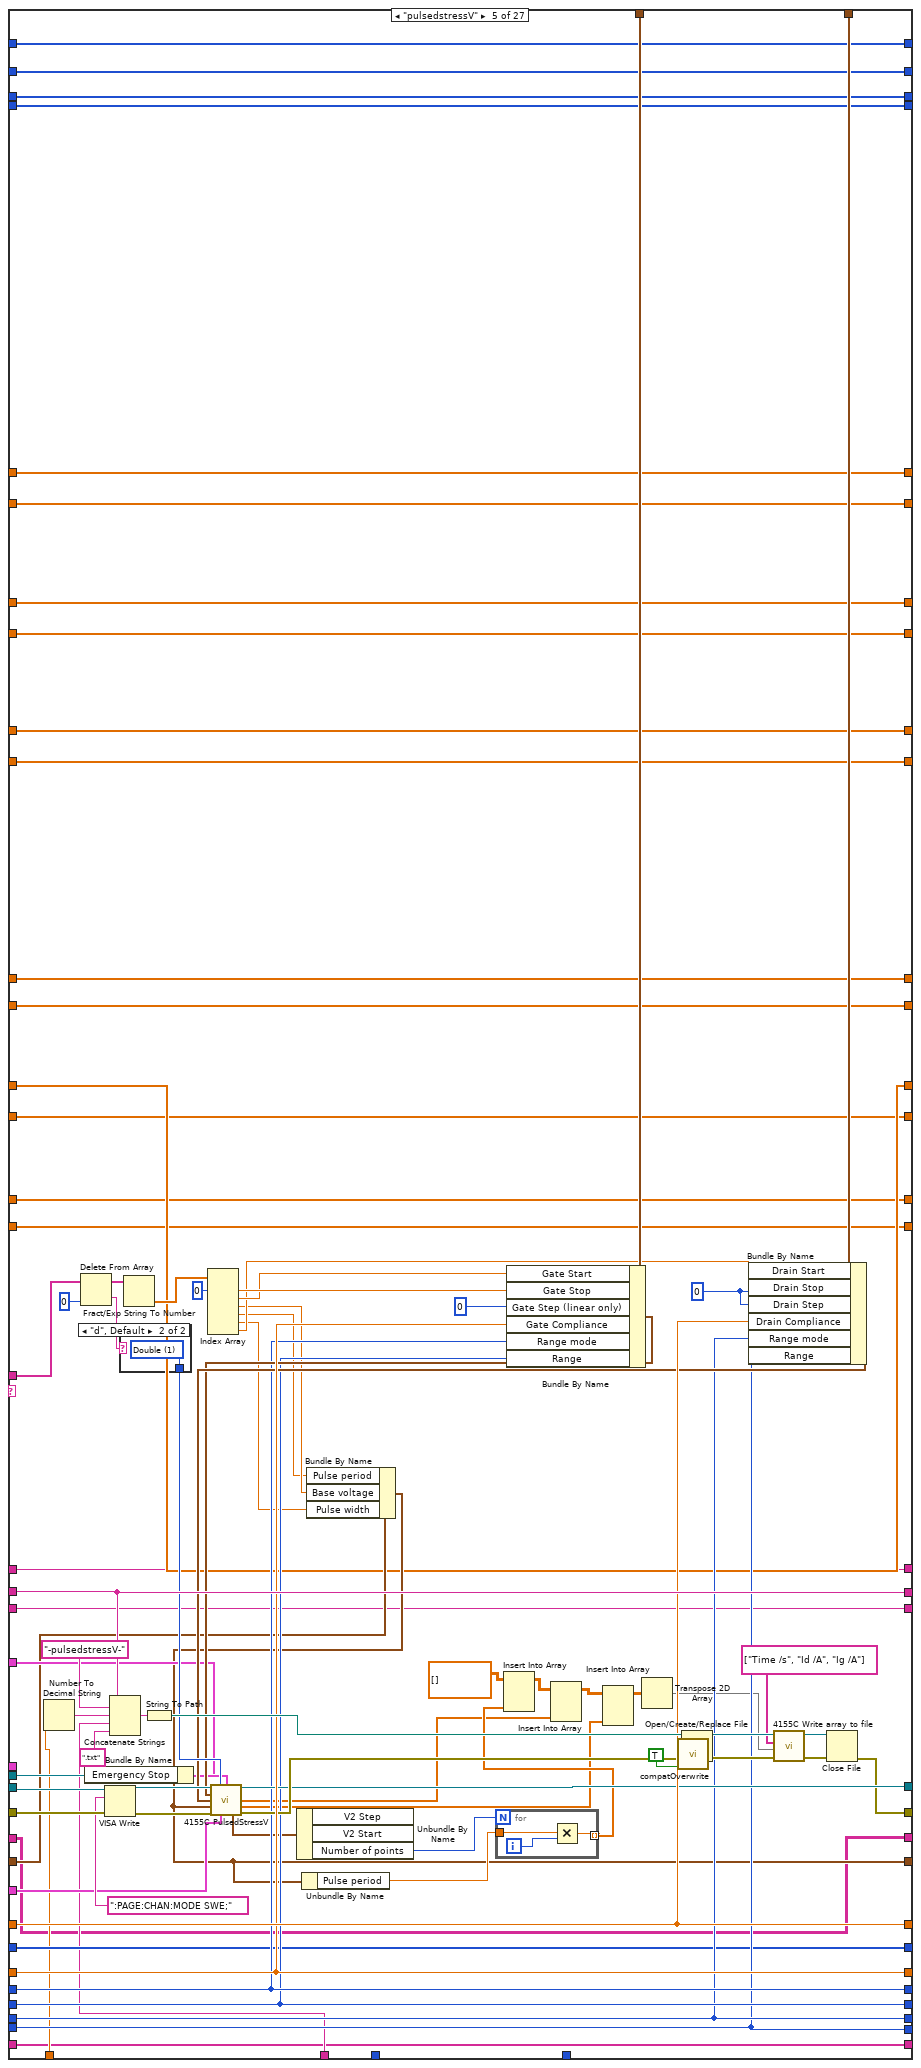
[diagram p10: hidden frame]
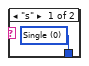
[diagram p11: hidden frame]
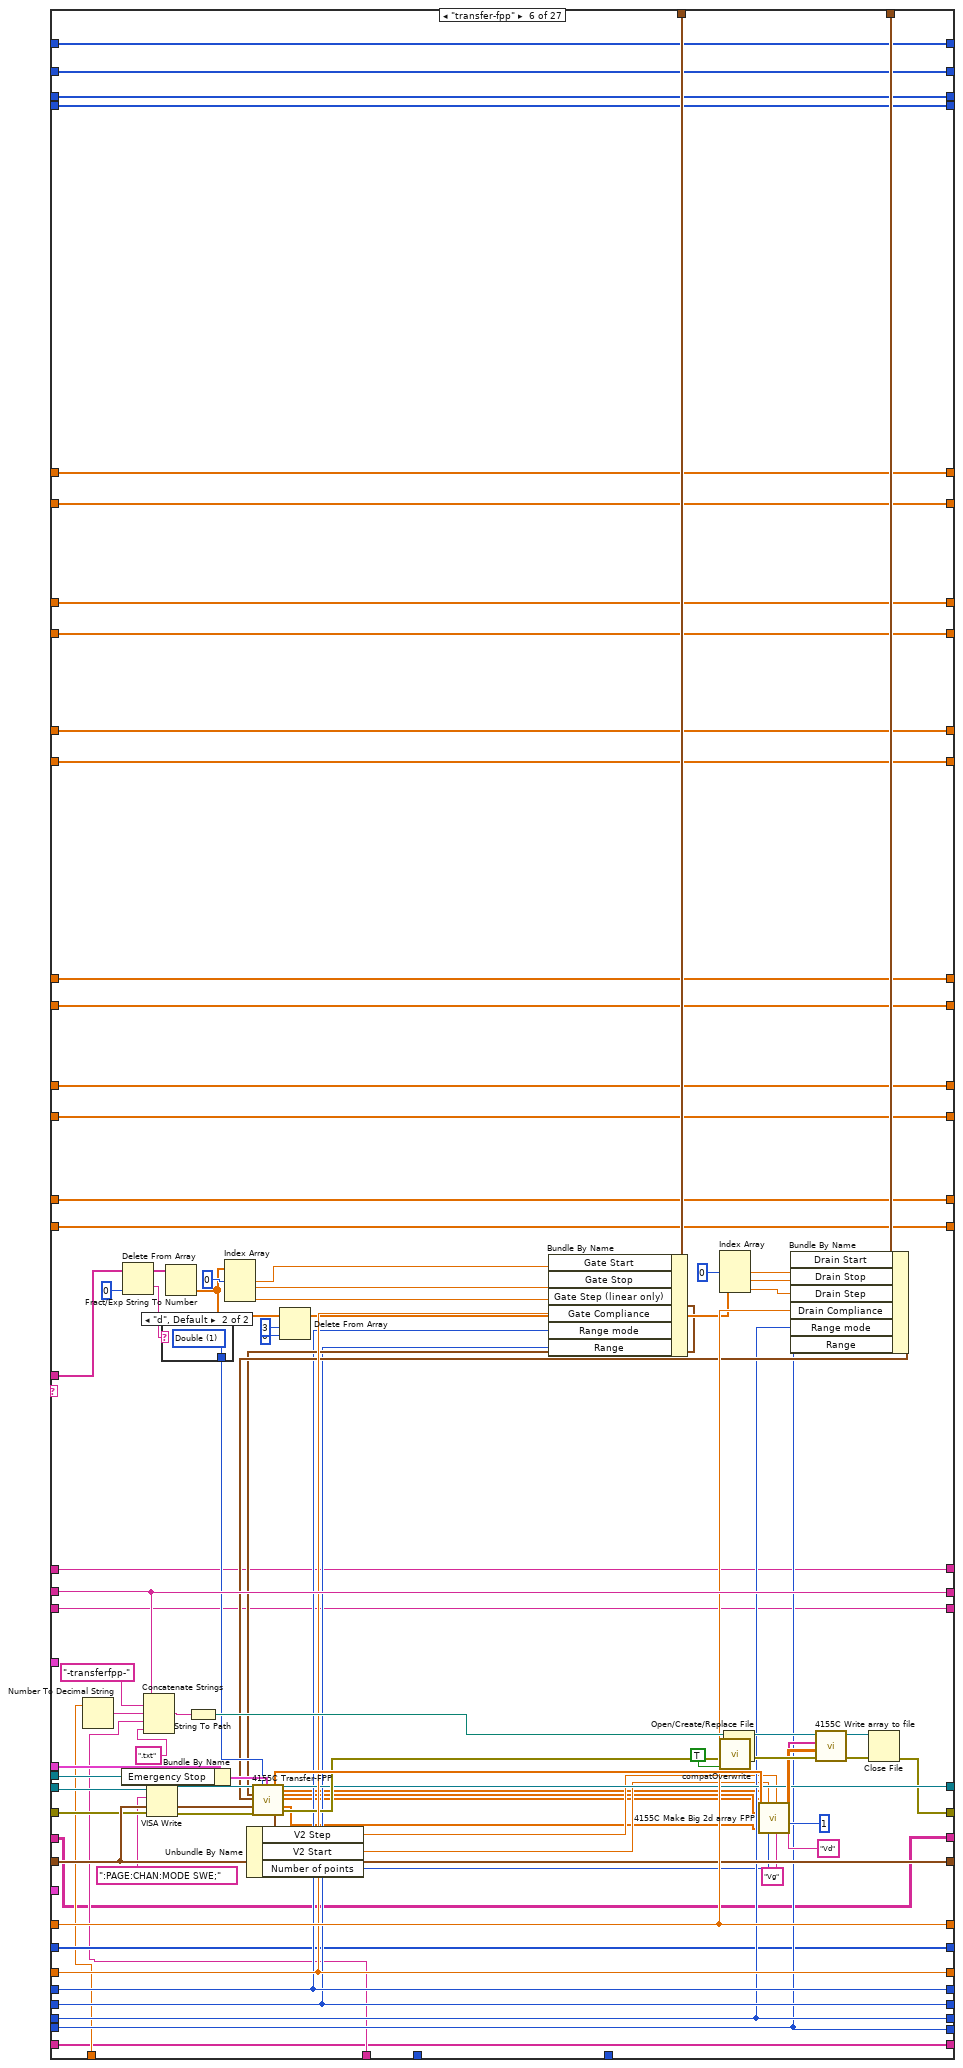
[diagram p12: hidden frame]
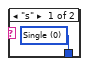
[diagram p13: hidden frame]
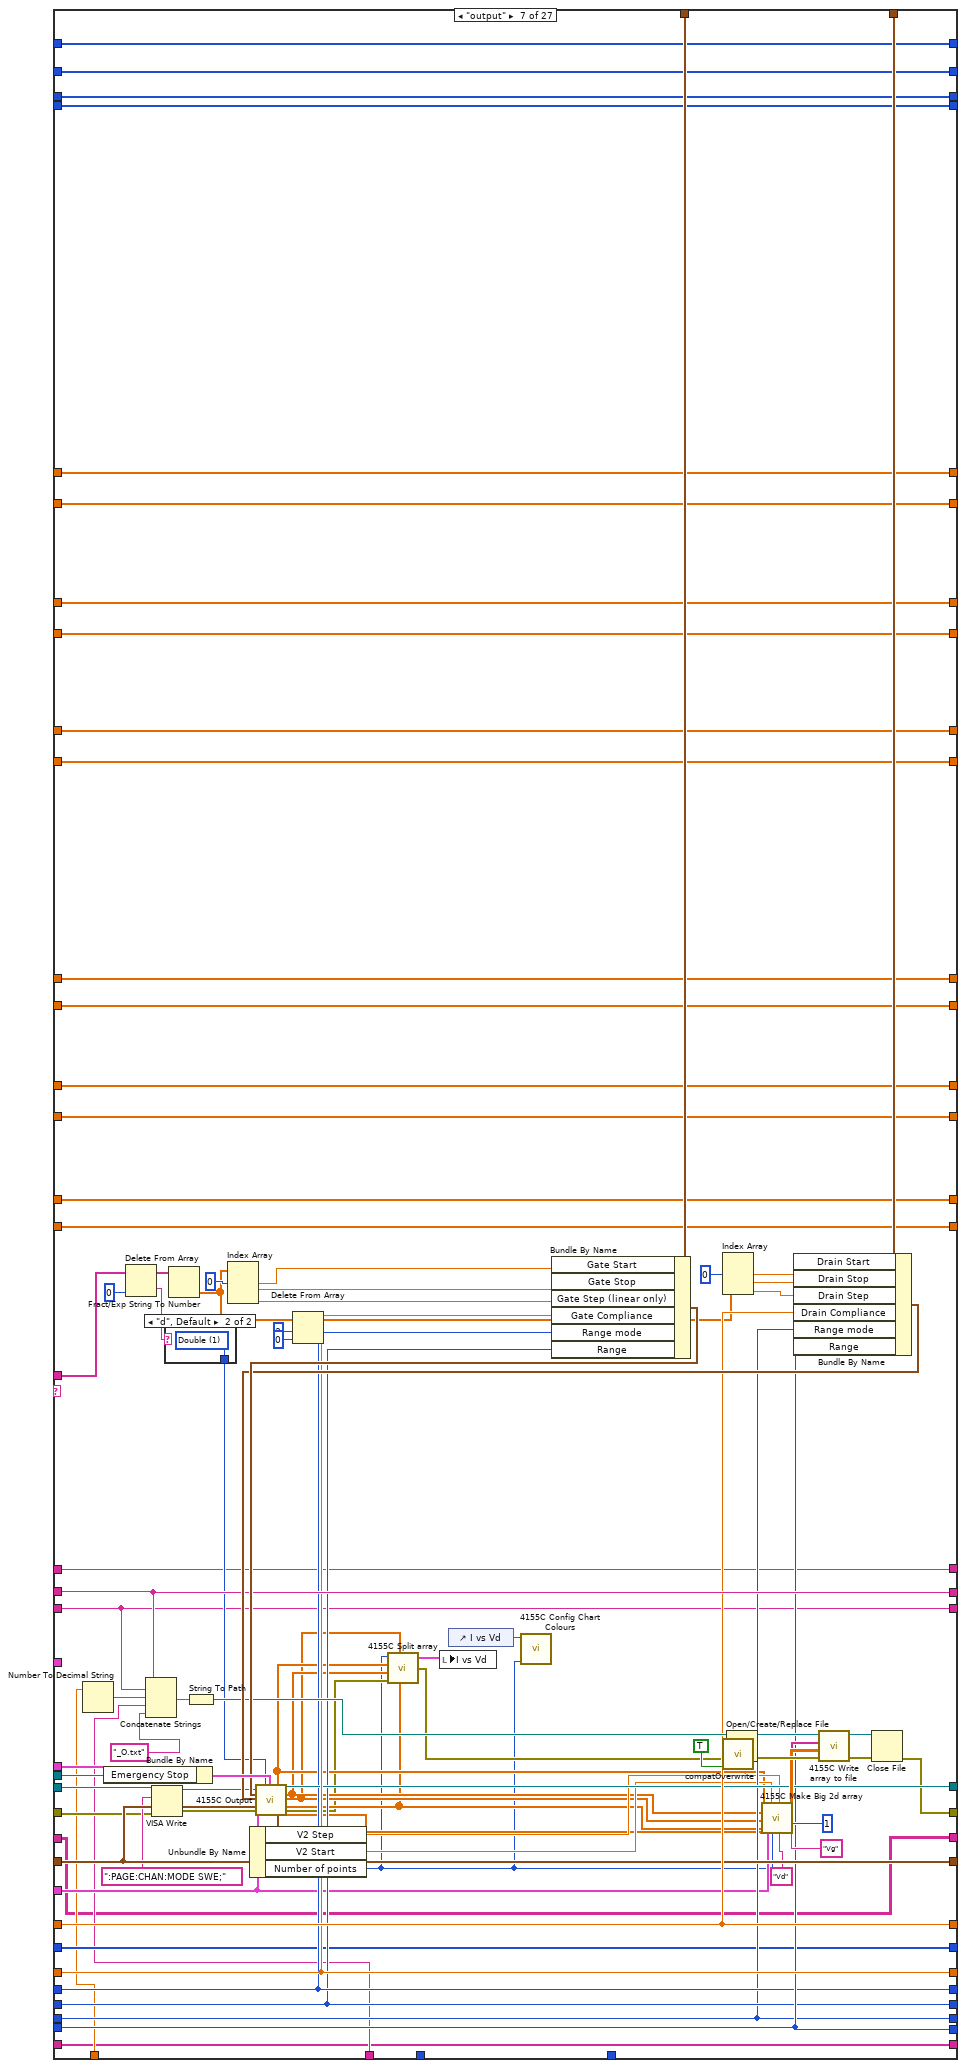
[diagram p14: hidden frame]
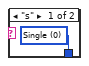
[diagram p15: hidden frame]
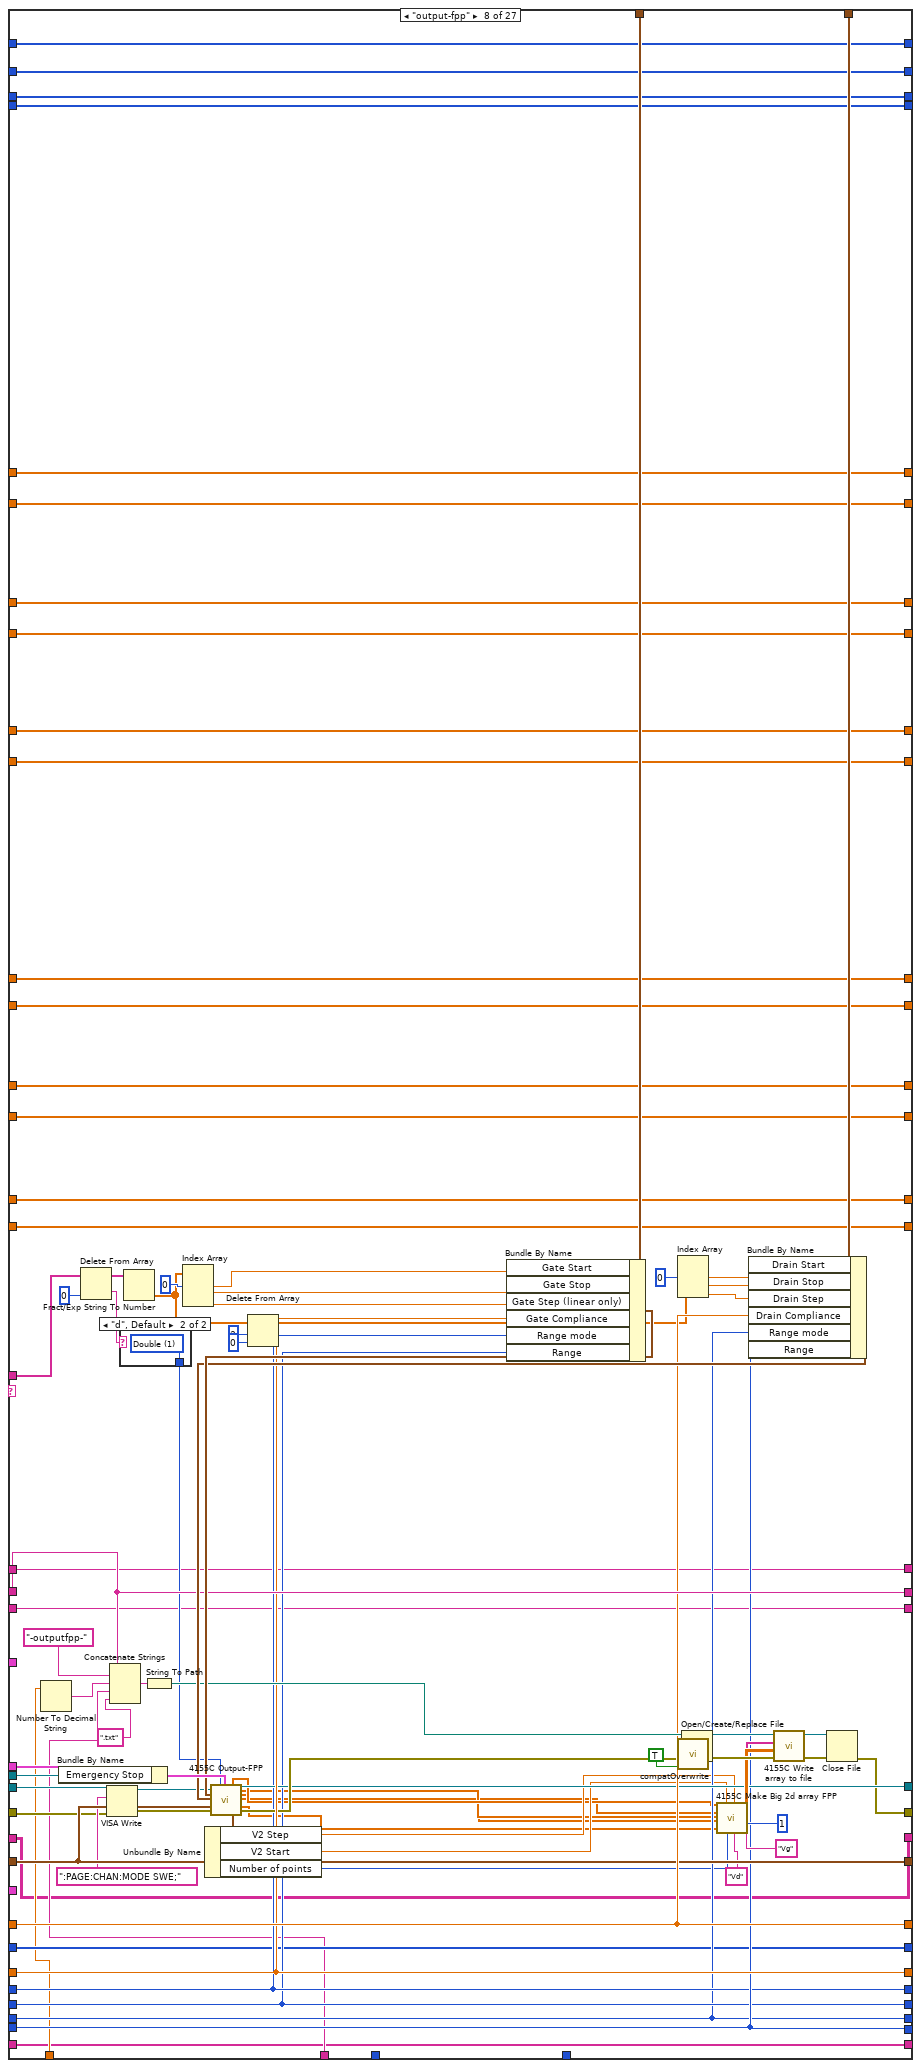
[diagram p16: hidden frame]
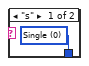
[diagram p17: hidden frame]
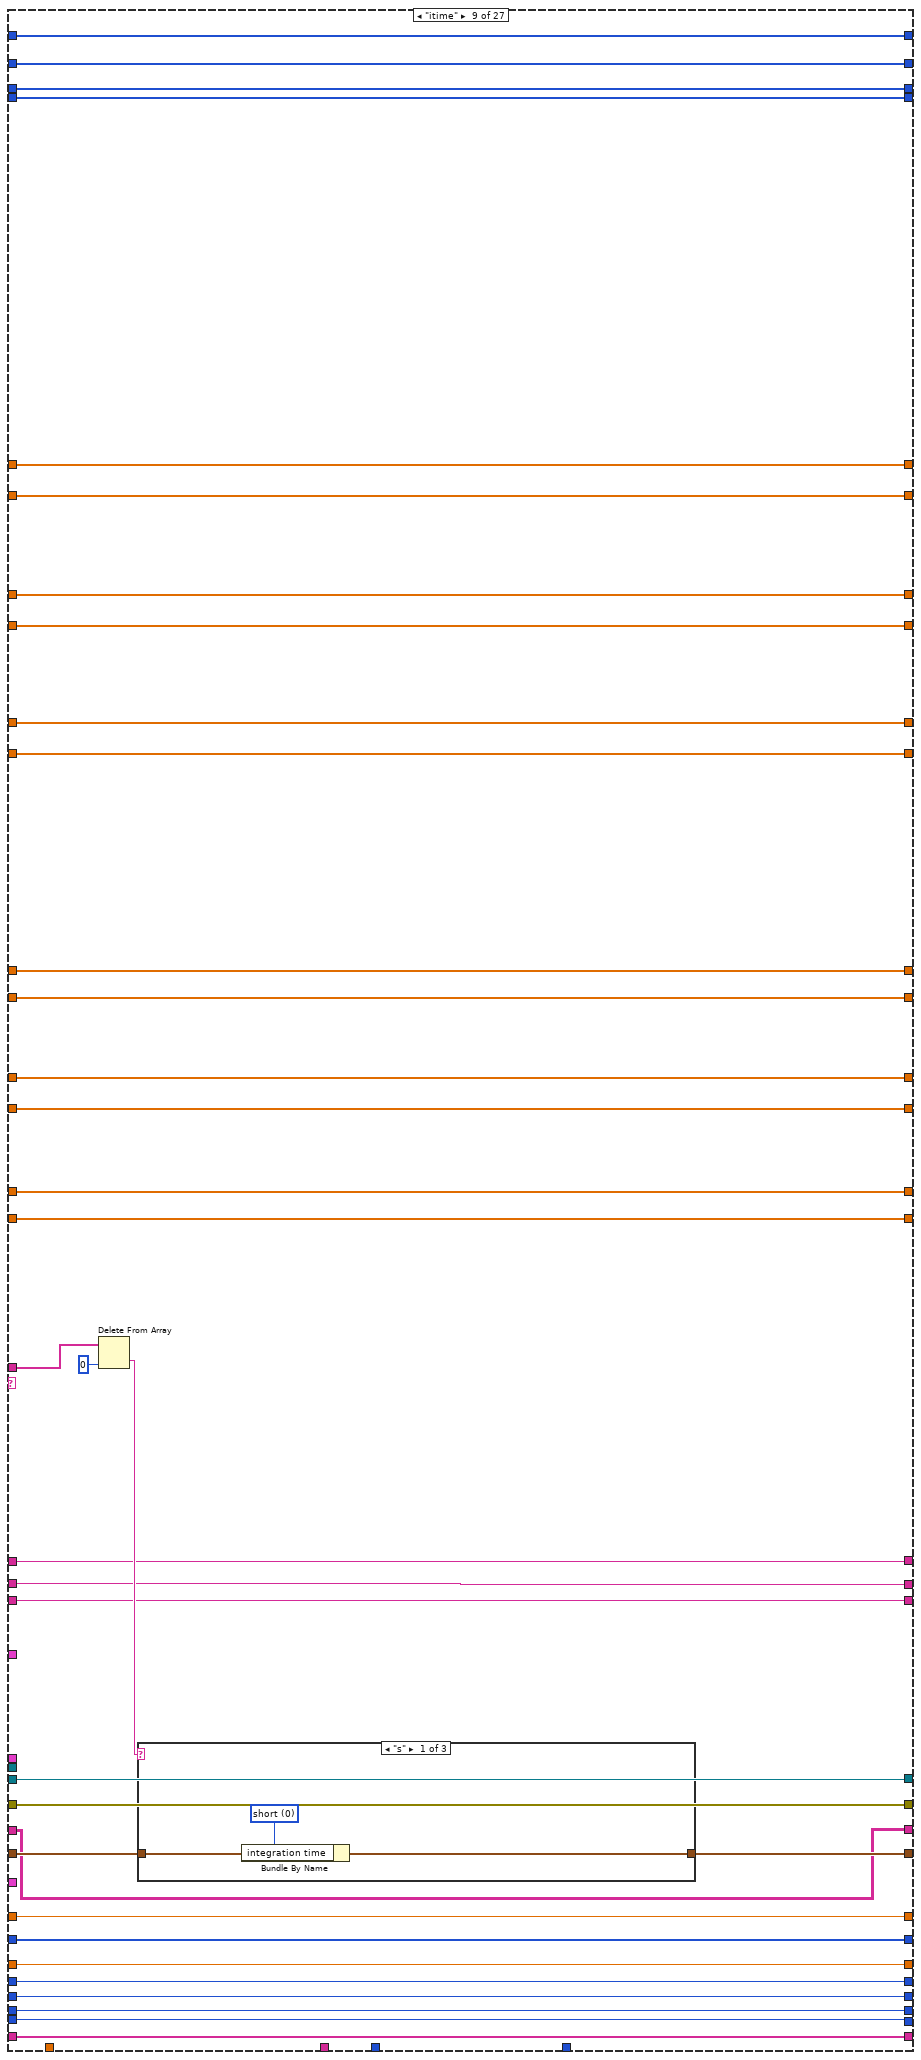
[diagram p18: hidden frame]
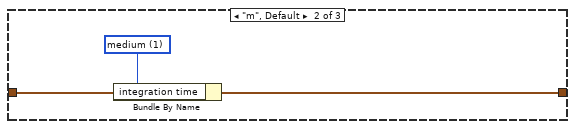
[diagram p19: hidden frame]
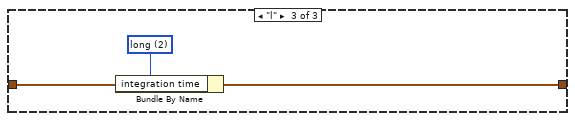
[diagram p20: hidden frame]
diagram:
  w49 = u16 1 items=["Reset All", "Partial reset"] ("Type of reset")
  # "Change from previous version:\n\n- Added array initialization."
  # "This is a version specific to the SPM pump."
  # "I add 1 to both the \"total lines\" and the \"line running\" indicators because i and N begin from 0, and the script lines begin from 1."
  # "Bugs:\n\n- If using the \"filename\" command, keep in mind that the arrays of the time-dependent data are not re-initialized inbetween filename changes. \n\n- Do not connect the \"error\" wire of a Split block if it has unconnected terminals! It will halt the program."
  # "Array size"
  # "%s option converts a spreadsheet string to an array of strings."
  # "0: No of rows of array\n1: No of cols"
  # "Dimitrios Simatos\nv. 5.4"
  # "Changes from original textcontrol.vi:\n\n- Timestamp appears in filename.\n- (Only) transfer and output curves are plotted.\n- Communication with serial port.\n- Can execute any command, as all pattern matching functions were replaced. Previously, commands with special LabVIEW characters could not be executed.\n- Replaced write to file function with write to text file.\n- Replaced while loop with for loop.\n- Replaced 4155C \"Save File\" function and now the vi can save time-dependent variables.\n- Added clock with start time control and various units.\n- Changed filepath in which the program is saved.\n- Added a serial output log that keeps a history.\n- Tab control.\n- Addition of specialized serial read/write file for the SPM OEM pump.\n- Added halt and hard stop.\n- Imax, Imin, Ion, and Ioff are now saved for all Is, Id, and Ig."
  # "Search and replace LF with EOL"
  n1 = Equal?(x="integration time", y=u32 0) -> (x = y?=w53:bool)
  n2 = Select(t="Integration time (short)", s=w53, f="Integration time (long)") -> (s? t:f=w57:dbl)
  n3 = call "4155C Get Filename.vi"("error in (no error)"=errorcluster {"status"=FALSE, "code"=0, "source"=""}) -> ("error out"=w44:errorcluster, "path"=w19:path)  [unwired: 2 in, 1 out]
  "Path" <- w19
  n4 = Bundle By Name(cluster="Timings 2", "integration time"="integration time", "Short/Long integration time"=w57, "hold time (sec)"="hold time /s", "delay time (sec)"="delay time /s", "Step Time (0 disables)"="Step delay /s") -> (w42:T6)
  n5 = Path To String(path=w19) -> (string=w20:string)
  n6 = Search and Replace String(replace all?=TRUE ("replace all? (F)"), input string="Script", search string="\n", replace string="\r\n") -> (result string=w32:string)  [unwired: 4 in, 3 out]
  n7 = Match Pattern(string=w20, regular expression=".txt") -> (before substring=w15:string)  [unwired: 1 in, 3 out]
  n8 = Concatenate Strings(w15, "Suffix (script)") -> (w14:string)
  n9 = call "4155C Initialise.vi"("VISA resource name in"=refnum<visa-resource-name> "GPIB0::14::INSTR", "Reset"="Full Reset", "Type of reset"=w49, "error in (no error)"=w44, "VISA Timeout Value"=u32 10000) -> ("VISA Resource Name out"=w43:refnum<visa-resource-name>, "error out"=w12:errorcluster)
  n10 = Spreadsheet String To Array(delimiter (Tab)="\r\n", format string="%s", spreadsheet string="Script", array type (2D Dbl)="") -> (array=w23:string[][])
  n11 = Array Size(array=w23) -> (size(s)=w27:i32[])
  n12 = Initialize Array("") -> (w4:string[])  [unwired: 1 in]
  n13 = String To Path(string=w14) -> (path=w13:path)
  n14 = Initialize Array(0 ("element")) -> (w6:i32[])  [unwired: 1 in]
  n15 = Initialize Array("") -> (w2:string[][])  [unwired: 2 in]
  n16 = Initialize Array(0.0 ("element")) -> (w8:dbl[])  [unwired: 1 in]
  n17 = Index Array(array=w27, index=0) -> (element=w25:i32)
  n18 = Write to Text File(file (use dialog)=w13, text=w32, error in=w12) -> (error out=w11:errorcluster)  [unwired: 1 in, 2 out]
  n19 = for {
    N: w25 -> [w167]
    tunnel: "SMU4" -> [w203]
    shift-left: "Source/Drain Range" -> [w208]
    shift-right: [w204] -> _
    shift-left: "Source/Drain\nRange mode" -> [w209]
    shift-right: [w205] -> _
    shift-left: "Gate Range" -> [w210]
    shift-right: [w206] -> _
    shift-left: "Gate Range\nmode" -> [w211]
    shift-right: [w207] -> _
    shift-left: "Gate: Compliance" -> [w220]
    shift-right: [w216] -> _
    shift-left: "Drain: Compliance" -> [w221]
    shift-right: [w217] -> _
    shift-left: w42 -> [w222]
    shift-right: [w218] -> _
    shift-left: w11 -> [w223]
    shift-right: [w113] -> w18
    shift-left: w43 -> [w224]
    shift-right: [w219] -> _
    shift-left: w15 -> [w225]
    shift-right: [w117] -> _
    tunnel: "Panel Controls 2" -> [w202]
    shift-right: [w75] -> _
    shift-left: w8 -> [w201]
    shift-right: [w137] -> _
    shift-left: _ -> [w197]
    tunnel: w23 -> [w196] mode=indexing
    shift-right: [w74] -> _
    shift-left: w8 -> [w173]
    shift-right: [w107] -> _
    shift-left: w4 -> [w159]
    shift-right: [w138] -> _
    shift-left: w6 -> [w154]
    shift-right: [w119] -> _
    shift-left: w6 -> [w153]
    shift-right: [w152] -> _
    shift-left: "" -> [w151]
    shift-right: [w112] -> _
    shift-left: w6 -> [w134]
    shift-right: [w111] -> _
    shift-left: w6 -> [w118]
    shift-right: [w108] -> _
    shift-left: w2 -> [w110]
    shift-right: [w68] -> _
    shift-left: w8 -> [w96]
    shift-right: [w69] -> _
    shift-left: w8 -> [w95]
    shift-right: [w73] -> _
    shift-left: w8 -> [w84]
    shift-right: [w72] -> _
    shift-left: w8 -> [w83]
    shift-right: [w66] -> _
    shift-left: w8 -> [w82]
    shift-right: [w76] -> _
    shift-left: w8 -> [w81]
    shift-right: [w67] -> _
    shift-left: w8 -> [w80]
    shift-right: [w65] -> _
    shift-left: w8 -> [w79]
    shift-right: [w71] -> _
    shift-left: w8 -> [w78]
    shift-right: [w70] -> _
    shift-left: w8 -> [w77]
    shift-right: [w60] -> _
    shift-left: "Filename (variable part)" -> [w59]
    i -> [w162]
    w98 = "Time (Minutes)" ("element")
    # "Filename prefix"
    # "Is off"
    # "Is on"
    # "Ig off"
    # "Ig on"
    # "Is min"
    # "Is max"
    # "Ig min"
    # "Ig max"
    # "Id min"
    # "Id max"
    # "Id off"
    # "Id on"
    # "Pump status"
    # "Filepath and name"
    # "Pump status"
    # "Limit of command arguments (array columns). Raise if needed."
    # "Serial port data (string)"
    # "Serial port data (table)"
    # "Time array for valve position"
    # "Time array for absolute plunger position"
    # "Valve position"
    # "Absolute plunger position"
    # "Serial port data"
    # "For loop counter"
    # "<-----Equivalent to the 4155C \"Write\" subvi.----->"
    # "Headers"
    # "Save transfer curves in file."
    # "Filepath and name"
    # "Save time-dependent data."
    # "Use the time offset if your measurements do not start at t=0."
    # "Time for Imax, Imin, Ion, Ioff"
    # "Rest of elements of command"
    # "First element of command\n(case select)"
    n20 = Add(x=w162, y=1) -> (x+y=→"Line running":i32)
    n21 = Add(x=w167, y=1) -> (x+y=→"Total lines":i32)
    n22 = Index Array(array=w196, index=0 ("line index")) -> (element=w191:string)
    "Command running:" <- w191
    n23 = control-ref of="Interrupt run"() -> (w215:refnum<vi>)
    n24 = Spreadsheet String To Array(delimiter (Tab)=" ", format string="%s", spreadsheet string=w191, array type (2D Dbl)=string[] []) -> (array=w189:string[])
    n25 = Delete From Array(array=w189, index=0) -> (deleted portion=w97:string, array with subset deleted=w188:string[])  [unwired: 1 in]
    n26 = call "Elapsed Time"("Reset"="Reset", "Auto Reset"="Auto Reset") -> ("Elapsed Time (s)"=w198:dbl)  [unwired: 10 in, 7 out]
    n27 = case shown="0, Default" "Units" {
      tunnel: ["_sec" "_min" "_h"] -> w199
      tunnel: [w226 w230 w233] -> w169
      tunnel: w198 -> [w226 w229 w234]
      frame 0, Default {
      }
      frame 1 {
        n28 = Divide(x=w229, y=60.0) -> (x/y=w230:dbl)
      }
      frame 2 {
        n29 = Divide(x=w234, y=3600.0) -> (x/y=w233:dbl)
      }
    }
    n30 = Add(x=w169, y="Time Offset") -> (x+y=w168:dbl)
    n31 = To Long Integer(number=w168) -> (32bit integer=w135:i32)
    "Elapsed Time" <- w135
    n32 = case shown="\"filename\"" w97 {
      tunnel: w188 -> [w271 w309 w346 w478 w502 w648 w742 w830 w887 w932 w978 w1022 w1062 w1095 _ _ w1256 w1336 _ w1439 w1502 w1563 w1652 w1733 w1772 w1842 w1896]
      tunnel: w225 -> [w266 w305 w344 w485 w567 w656 w749 w838 w876 w921 w970 w1015 w1056 w1088 w1126 w1187 w1234 w1318 w1368 w1426 w1489 w1551 w1646 w1729 w1774 w1844 w1898]
      tunnel: w224 -> [w265 w304 w335 w456 w552 w625 w718 w806 w877 w922 w971 w1016 w1057 w1089 w1131 w1189 w1262 w1342 w1372 w1445 w1508 w1569 w1658 w1687 w1778 w1848 w1900]
      tunnel: w223 -> [w264 w303 w334 w455 w551 w624 w715 w803 w878 w923 w972 w1017 w1058 w1090 w1130 w1160 w1261 w1341 w1371 w1444 w1507 w1568 w1657 w1686 w1777 w1847 w1901]
      tunnel: w222 -> [w263 w302 w343 w481 w527 w652 w745 w834 w886 w931 w969 w1014 w1055 w1087 w1129 w1184 w1225 w1310 w1377 w1419 w1482 w1544 w1645 w1728 w1779 w1849 w1903]
      tunnel: w221 -> [w262 w301 w342 w483 w565 w654 w747 w836 w885 w930 w977 w1021 w1061 w1094 w1128 w1169 w1260 w1340 w1380 w1443 w1506 w1567 w1656 w1737 w1780 w1850 w1904]
      tunnel: w220 -> [w261 w300 w341 w482 w564 w653 w746 w835 w884 w929 w976 w1020 w1060 w1093 w1127 w1170 w1235 w1319 w1379 w1427 w1490 w1552 w1647 w1730 w1782 w1851 w1906]
      tunnel: [w265 w304 w333 w480 w562 w650 w744 w832 w877 w922 w971 w1016 w1057 w1089 w1131 w1189 w1226 w1292 w1370 w1420 w1483 w1545 w1598 w1689 w1778 w1848 w1900] -> w219
      tunnel: [w264 w303 w332 w479 w561 w649 w743 w831 w878 w923 w972 w1017 w1058 w1090 w1130 w1159 w1236 w1293 w1369 w1428 w1491 w1553 w1597 w1688 w1776 w1846 w1901] -> w133
      tunnel: [w263 w302 w343 w481 w523 w652 w745 w834 w879 w924 w969 w1014 w1055 w1087 w1129 w1184 w1225 w1310 w1377 w1419 w1482 w1544 w1645 w1728 w1779 w1849 w1903] -> w218
      tunnel: [w262 w301 w342 w483 w565 w654 w747 w836 w885 w930 w977 w1021 w1061 w1094 w1128 w1169 w1260 w1340 w1380 w1443 w1506 w1567 w1656 w1737 w1780 w1850 w1904] -> w217
      tunnel: [w261 w300 w341 w482 w564 w653 w746 w835 w884 w929 w976 w1020 w1060 w1093 w1127 w1170 w1235 w1319 w1379 w1427 w1490 w1552 w1647 w1730 w1782 w1851 w1906] -> w216
      tunnel: [w266 w305 w344 w485 w567 w656 w749 w838 w876 w921 w970 w1015 w1056 w1088 w1126 w1187 w1234 w1318 w1368 w1426 w1489 w1551 w1646 w1729 w1774 w1844 w1898] -> w117
      tunnel: w215 -> [_ _ _ w487 w571 w661 w752 w842 _ _ _ _ _ _ _ _ w1231 w1315 _ w1425 w1488 w1550 w1618 w1705 _ _ _]
      tunnel: "Gate" -> [_ _ _ w465 w555 w635 w729 w817 _ _ _ _ _ _ _ _ _ _ _ _ _ _ _ _ _ _ _]
      tunnel: "Drain 2" -> [_ _ _ w464 w554 w634 w728 w816 _ _ _ _ _ _ _ _ _ _ _ _ _ _ _ _ _ _ _]
      tunnel: "Panel Controls" -> [_ _ _ _ _ w633 w727 w815 _ _ _ _ _ _ _ _ _ _ _ _ _ _ _ _ _ _ _]
      tunnel: w211 -> [w260 w299 w340 w449 w545 w618 w713 w801 w883 w928 _ w1013 w1054 w1086 w1125 w1171 w1221 w1306 w1373 w1415 w1478 w1540 w1641 w1724 w1783 w1852 w1907]
      tunnel: w210 -> [w259 w298 w339 w448 w544 w617 w712 w800 w882 w927 w975 _ w1045 w1092 w1124 w1172 w1222 w1307 w1374 w1416 w1479 w1541 w1642 w1725 w1784 w1853 w1908]
      tunnel: w209 -> [w258 w297 w338 w447 w543 w616 w711 w799 w881 w926 w974 w1019 w1059 _ w1123 w1173 w1223 w1308 w1375 w1417 w1480 w1542 w1643 w1726 w1785 w1854 w1909]
      tunnel: w208 -> [w257 w296 w337 w446 w542 w615 w714 w802 w880 w925 w973 w1018 _ w1091 w1122 w1174 w1224 w1309 w1376 w1418 w1481 w1543 w1644 w1727 w1786 w1855 w1910]
      tunnel: [w260 w299 w340 w449 w545 w618 w713 w801 w883 w928 w968 w1013 w1054 w1086 w1125 w1171 w1221 w1306 w1373 w1415 w1478 w1540 w1641 w1724 w1783 w1852 w1907] -> w207
      tunnel: [w259 w298 w339 w448 w544 w617 w712 w800 w882 w927 w975 w1005 w1045 w1092 w1124 w1172 w1222 w1307 w1374 w1416 w1479 w1541 w1642 w1725 w1784 w1853 w1908] -> w206
      tunnel: [w258 w297 w338 w447 w543 w616 w711 w799 w881 w926 w974 w1019 w1059 w1085 w1123 w1173 w1223 w1308 w1375 w1417 w1480 w1542 w1643 w1726 w1785 w1854 w1909] -> w205
      tunnel: [w257 w296 w337 w446 w542 w615 w714 w802 w880 w925 w973 w1018 w1046 w1091 w1122 w1174 w1224 w1309 w1376 w1418 w1481 w1543 w1644 w1727 w1786 w1855 w1910] -> w204
      tunnel: w203 -> [_ _ _ w441 w539 _ w707 _ _ _ _ _ _ _ _ _ _ _ _ _ _ _ _ _ _ _ _]
      tunnel: w202 -> [_ _ _ w439 w538 _ _ _ _ _ _ _ _ _ _ _ _ _ _ _ _ _ _ _ _ _ _]
      tunnel: [w256 w292 w330 w367 w515 w605 w704 w788 w875 w919 w967 w1004 w1044 w1084 w1121 w1155 w1213 w1271 w1367 w1404 w1471 w1534 w1595 w1682 w1775 w1845 w1915] -> w75
      tunnel: w201 -> [w256 w292 w330 w436 w515 w605 w704 w788 w875 w919 w967 w1004 w1044 w1084 w1121 w1155 w1213 w1271 w1367 w1404 w1471 w1534 w1595 w1682 w1775 w1845 w1915]
      tunnel: w168 -> [_ _ _ w433 w512 w603 w701 w785 _ _ _ _ _ _ _ w1153 w1211 w1288 _ w1401 w1468 w1531 w1592 w1678 _ _ _]
      tunnel: w199 -> [_ _ _ w430 w511 w601 w700 w784 _ _ _ _ _ _ _ w1151 w1209 w1287 _ w1400 w1467 w1530 w1591 w1679 _ w1813 _]
      tunnel: w135 -> [_ _ _ w425 _ _ _ _ _ _ _ _ _ _ _ _ _ _ _ _ _ _ _ _ _ w1816 _]
      tunnel: [w255 w291 w329 w375 w514 w604 w703 w787 w874 w918 w966 w1003 w1043 w1083 w1120 w1154 w1212 w1290 w1366 w1403 w1470 w1533 w1594 w1681 w1781 w1825 w1905] -> w137
      tunnel: w197 -> [w255 w291 w329 w429 w514 w604 w703 w787 w874 w918 w966 w1003 w1043 w1083 w1120 w1154 w1212 w1290 w1366 w1403 w1470 w1533 w1594 w1681 w1781 w1825 w1905]
      tunnel: [w254 w290 w328 w366 w510 w600 w699 w783 w873 w917 w965 w1002 w1042 w1082 w1119 w1150 w1208 w1270 w1365 w1399 w1466 w1529 w1590 w1677 w1770 w1841 w1914] -> w74
      tunnel: w173 -> [w254 w290 w328 w423 w510 w600 w699 w783 w873 w917 w965 w1002 w1042 w1082 w1119 w1150 w1208 w1270 w1365 w1399 w1466 w1529 w1590 w1677 w1770 w1841 w1914]
      tunnel: [w253 w289 w327 w416 w509 w599 w689 w782 w872 w916 w964 w1001 w1041 w1081 w1118 w1149 w1207 w1286 w1364 w1398 w1465 w1528 w1589 w1676 w1769 w1840 w1911] -> w107
      tunnel: w159 -> [w253 w289 w327 w416 w509 w599 w689 w782 w872 w916 w964 w1001 w1041 w1081 w1118 w1149 w1207 w1286 w1364 w1398 w1465 w1528 w1589 w1676 w1768 w1814 w1911]
      tunnel: [w252 w288 w326 w415 w508 w598 w688 w781 w871 w915 w963 w1000 w1040 w1080 w1117 w1148 w1206 w1285 w1363 w1397 w1464 w1527 w1588 w1675 w1754 w1827 w1925] -> w138
      tunnel: w154 -> [w252 w288 w326 w415 w508 w598 w688 w781 w871 w915 w963 w1000 w1040 w1080 w1117 w1148 w1206 w1285 w1363 w1397 w1464 w1527 w1588 w1675 w1754 w1826 w1925]
      tunnel: [w251 w287 w325 w414 w507 w597 w687 w780 w870 w914 w962 w999 w1039 w1079 w1116 w1147 w1205 w1284 w1362 w1396 w1463 w1526 w1587 w1674 w1753 w1809 w1927] -> w119
      tunnel: w153 -> [w251 w287 w325 w414 w507 w597 w687 w780 w870 w914 w962 w999 w1039 w1079 w1116 w1147 w1205 w1284 w1362 w1396 w1463 w1526 w1587 w1674 w1753 w1807 w1927]
      tunnel: [w250 w286 w324 w413 w506 w596 w686 w779 w869 w913 w961 w998 w1038 w1078 w1115 w1146 w1204 w1283 w1361 w1395 w1462 w1525 w1586 w1673 w1752 w1806 w1899] -> w152
      tunnel: w151 -> [w250 w286 w324 w413 w506 w596 w686 w779 w869 w913 w961 w998 w1038 w1078 w1115 w1146 w1204 w1283 w1361 w1395 w1462 w1525 w1586 w1673 w1752 w1817 w1899]
      tunnel: w135 -> [_ _ _ _ _ _ _ _ _ _ _ _ _ _ _ _ _ _ _ _ _ _ _ _ _ w1805 _]
      tunnel: w134 -> [w249 w285 w323 w412 w505 w595 w685 w778 w868 w912 w960 w997 w1037 w1077 w1114 w1145 w1203 w1282 w1360 w1394 w1461 w1524 w1585 w1672 w1751 w1804 w1926]
      tunnel: [w249 w285 w323 w412 w505 w595 w685 w778 w868 w912 w960 w997 w1037 w1077 w1114 w1145 w1203 w1282 w1360 w1394 w1461 w1524 w1585 w1672 w1751 w1803 w1926] -> w112
      tunnel: [w248 w284 w322 w411 w504 w594 w684 w777 w867 w911 w959 w996 w1036 w1076 w1113 w1144 w1202 w1281 w1359 w1393 w1460 w1523 w1584 w1671 w1750 w1802 w1924] -> w111
      tunnel: w118 -> [w248 w284 w322 w411 w504 w594 w684 w777 w867 w911 w959 w996 w1036 w1076 w1113 w1144 w1202 w1281 w1359 w1393 w1460 w1523 w1584 w1671 w1750 w1801 w1924]
      tunnel: [w247 w283 w321 w410 w503 w593 w683 w776 w866 w910 w958 w995 w1035 w1075 w1112 w1143 w1201 w1280 w1358 w1392 w1459 w1522 w1583 w1670 w1749 w1799 w1902] -> w108
      tunnel: w110 -> [w247 w283 w321 w410 w503 w593 w683 w776 w866 w910 w958 w995 w1035 w1075 w1112 w1143 w1201 w1280 w1358 w1392 w1459 w1522 w1583 w1670 w1749 w1798 w1902]
      tunnel: [w245 w281 w319 w360 w500 w591 w681 w774 w864 w909 w957 w993 w1033 w1073 w1110 w1141 w1200 w1279 w1357 w1391 w1458 w1520 w1582 w1669 w1748 w1797 w1920] -> w68
      tunnel: w96 -> [w245 w281 w319 w406 w500 w591 w681 w774 w864 w909 w957 w993 w1033 w1073 w1110 w1141 w1200 w1279 w1357 w1391 w1458 w1520 w1582 w1669 w1748 w1797 w1920]
      tunnel: [w246 w282 w320 w361 w501 w592 w682 w775 w865 w908 w956 w994 w1034 w1074 w1111 w1142 w1199 w1278 w1356 w1390 w1457 w1521 w1581 w1668 w1747 w1796 w1921] -> w69
      tunnel: w95 -> [w246 w282 w320 w405 w501 w592 w682 w775 w865 w908 w956 w994 w1034 w1074 w1111 w1142 w1199 w1278 w1356 w1390 w1457 w1521 w1581 w1668 w1747 w1796 w1921]
      tunnel: [w238 w274 w312 w365 w497 w589 w679 w772 w857 w906 w954 w991 w1031 w1071 w1108 w1134 w1192 w1269 w1355 w1383 w1450 w1513 w1574 w1663 w1740 w1795 w1913] -> w73
      tunnel: w84 -> [w238 w274 w312 w395 w497 w589 w679 w772 w857 w906 w954 w991 w1031 w1071 w1108 w1134 w1192 w1269 w1355 w1383 w1450 w1513 w1574 w1663 w1740 w1795 w1913]
      tunnel: [w237 w273 w311 w364 w498 w590 w680 w773 w856 w907 w955 w992 w1032 w1072 w1109 w1133 w1191 w1268 w1354 w1382 w1449 w1512 w1573 w1662 w1739 w1794 w1912] -> w72
      tunnel: w83 -> [w237 w273 w311 w394 w498 w590 w680 w773 w856 w907 w955 w992 w1032 w1072 w1109 w1133 w1191 w1268 w1354 w1382 w1449 w1512 w1573 w1662 w1739 w1794 w1912]
      tunnel: [w240 w276 w314 w370 w496 w587 w677 w770 w862 w904 w952 w989 w1029 w1069 w1106 w1136 w1194 w1273 w1349 w1385 w1452 w1515 w1576 w1661 w1744 w1792 w1917] -> w66
      tunnel: w82 -> [w240 w276 w314 w391 w496 w587 w677 w770 w862 w904 w952 w989 w1029 w1069 w1106 w1136 w1194 w1273 w1349 w1385 w1452 w1515 w1576 w1661 w1744 w1792 w1917]
      tunnel: [w239 w275 w313 w368 w499 w588 w678 w771 w863 w905 w953 w990 w1030 w1070 w1107 w1135 w1193 w1272 w1348 w1384 w1451 w1514 w1575 w1660 w1743 w1793 w1916] -> w76
      tunnel: w81 -> [w239 w275 w313 w390 w499 w588 w678 w771 w863 w905 w953 w990 w1030 w1070 w1107 w1135 w1193 w1272 w1348 w1384 w1451 w1514 w1575 w1660 w1743 w1793 w1916]
      tunnel: [w242 w278 w316 w359 w495 w585 w675 w768 w860 w902 w950 w987 w1027 w1067 w1104 w1138 w1196 w1275 w1351 w1387 w1454 w1517 w1578 w1665 w1746 w1790 w1919] -> w67
      tunnel: w80 -> [w242 w278 w316 w387 w495 w585 w675 w768 w860 w902 w950 w987 w1027 w1067 w1104 w1138 w1196 w1275 w1351 w1387 w1454 w1517 w1578 w1665 w1746 w1790 w1919]
      tunnel: [w241 w277 w315 w358 w494 w586 w676 w769 w861 w903 w951 w988 w1028 w1068 w1105 w1137 w1195 w1274 w1350 w1386 w1453 w1516 w1577 w1664 w1745 w1791 w1918] -> w65
      tunnel: w79 -> [w241 w277 w315 w386 w494 w586 w676 w769 w861 w903 w951 w988 w1028 w1068 w1105 w1137 w1195 w1274 w1350 w1386 w1453 w1516 w1577 w1664 w1745 w1791 w1918]
      tunnel: [w244 w280 w318 w363 w493 w583 w673 w766 w858 w900 w948 w985 w1025 w1065 w1102 w1140 w1198 w1277 w1353 w1389 w1456 w1519 w1580 w1667 w1742 w1788 w1923] -> w71
      tunnel: w78 -> [w244 w280 w318 w383 w493 w583 w673 w766 w858 w900 w948 w985 w1025 w1065 w1102 w1140 w1198 w1277 w1353 w1389 w1456 w1519 w1580 w1667 w1742 w1788 w1923]
      tunnel: [w243 w279 w317 w362 w492 w584 w674 w767 w859 w901 w949 w986 w1026 w1066 w1103 w1139 w1197 w1276 w1352 w1388 w1455 w1518 w1579 w1666 w1741 w1789 w1922] -> w70
      tunnel: w77 -> [w243 w279 w317 w382 w492 w584 w674 w767 w859 w901 w949 w986 w1026 w1066 w1103 w1139 w1197 w1276 w1352 w1388 w1455 w1518 w1579 w1666 w1741 w1789 w1922]
      tunnel: w59 -> [w236 w272 w310 w349 w491 w582 w672 w765 w855 w899 w947 w984 w1024 w1064 w1101 w1132 w1190 w1267 w1347 w1381 w1448 w1511 w1572 w1659 w1738 w1787 _]
      tunnel: [w236 w272 w310 w349 w491 w582 w672 w765 w855 w899 w947 w984 w1024 w1064 w1101 w1132 w1190 w1267 w1347 w1381 w1448 w1511 w1572 w1659 w1738 w1787 w1895] -> w60
      frame "wait" {
        n33 = Index Array(array=w271, index=0 ("Index")) -> (element=w269:string)
        n34 = Decimal String To Number(string=w269, default (0L)=u32 0) -> (number=w268:u32)  [unwired: 1 in, 1 out]
        n35 = Wait (ms)(milliseconds to wait=w268) -> ()  [unwired: 1 out]
      }
      frame "wait-min" {
        n36 = Index Array(array=w309, index=0 ("Index")) -> (element=w307:string)
        n37 = Decimal String To Number(string=w307, default (0L)=u32 0) -> (number=w295:u32)  [unwired: 1 in, 1 out]
        n38 = Multiply(x=w295, y=u32 60000) -> (x*y=w294:u32)
        n39 = Wait (ms)(milliseconds to wait=w294) -> ()  [unwired: 1 out]
      }
      frame "standby" {
        n40 = Index Array(array=w346, index=0 ("Index")) -> (element=w336:string)
        n41 = case shown="\"off\", Default" w336 {
          tunnel: [":PAGE:SCON:STAN 0" ":PAGE:SCON:STAN 1"] -> w331
          frame "off", Default {
          }
          frame "on" {
          }
        }
        n42 = VISA Write(VISA resource name=w335, write buffer=w331, error in (no error)=w334) -> (VISA resource name out=w333:refnum<visa-resource-name>, error out=w332:errorcluster)  [unwired: 1 out]
      }
      frame "transfer" {
        # "Adjusts graph colors."
        # "Adjusts graph colors."
        # "Is off"
        # "Is on"
        # "Ion will be the middle element of the array. The calculation of the index is done only once, since Is, Id, and Ig have the same dimensions."
        # "Ig off"
        # "Ig on"
        # "Is min"
        # "Is max"
        # "Ig min"
        # "Ig max"
        # "abs(Ig)"
        # "abs(Is)"
        # "Id min"
        # "Id max"
        # "Y1: Is\nY2: Id\nY3: Ig"
        # "abs(Id)"
        # "Adjusts graph colors."
        # "Adjusts graph colors."
        # "Id off"
        # "Id on"
        # "Don't connect the error lines\nof the two Split blocks!"
        # "Adjusts graph colors."
        # "Time array"
        n43 = Delete From Array(array=w478, index=0 ("Index")) -> (deleted portion=w476:string, array with subset deleted=w475:string[])  [unwired: 1 in]
        n44 = Bundle By Name(cluster=w439, "Emergency Stop"=w487) -> (w440:T2)
        n45 = Number To Decimal String(number=w433) -> (decimal integer string=w432:string)  [unwired: 1 in]
        n46 = case shown="\"d\", Default" w476 {
          tunnel: [w489 w490] -> w474
          frame "s" {
            w489 = u16 0 items=["Single", "Double"] ("sweep mode")
          }
          frame "d", Default {
            w490 = u16 1 items=["Single", "Double"] ("sweep mode")
          }
        }
        n47 = Fract/Exp String To Number(string=w475) -> (number=w460:dbl[])  [unwired: 3 in, 1 out]
        n48 = Concatenate Strings(w485, w349, w432, w430, "_T.txt" ("Suffix (transfer)")) -> (w486:string)
        n49 = VISA Write(VISA resource name=w456, write buffer=":PAGE:CHAN:MODE SWE;" ("write buffer (\"\")"), error in (no error)=w455) -> (VISA resource name out=w453:refnum<visa-resource-name>, error out=w454:errorcluster)  [unwired: 1 out]
        n50 = String To Path(string=w486) -> (path=w484:path)
        n51 = Index Array(array=w460, index #1=0 ("Index")) -> (element #1=w473:dbl, element #2=w472:dbl, element #3=w471:dbl)  [unwired: 2 in]
        n52 = Delete From Array(array=w460, length=3 ("Length"), index=0 ("Index")) -> (array with subset deleted=w458:dbl[])  [unwired: 1 out]
        n53 = Build Array (concatenate)(w429, w425) -> (w375:i32[])
        n54 = Bundle By Name(cluster=w465, "Gate Start"=w473, "Gate Stop"=w472, "Gate Step (linear only)"=w471, "Gate Compliance"=w482, "Range mode"=w449, "Range"=w448) -> (w450:T4)
        n55 = control-ref of="Imax vs time"() -> (w404:refnum<vi>)
        n56 = control-ref of="Imin vs time"() -> (w403:refnum<vi>)
        n57 = control-ref of="Ion vs time"() -> (w372:refnum<vi>)
        n58 = control-ref of="Ioff vs time"() -> (w371:refnum<vi>)
        n59 = control-ref of="I vs Vg"() -> (w434:refnum<vi>)
        n60 = Index Array(array=w458, index #1=0 ("Index")) -> (element #1=w468:dbl, element #2=w467:dbl, element #3=w466:dbl)  [unwired: 2 in]
        n61 = call <vilib>:"compatOverwrite.vi"("overwrite (F)"=TRUE) -> ("overwrite?"=w438:T7)
        n62 = Bundle By Name(cluster=w464, "Drain Start"=w468, "Drain Stop"=w467, "Drain Step"=w466, "Drain Compliance"=w483, "Range mode"=w447, "Range"=w446) -> (w451:T5)
        n63 = call "4155C Transfer.vi"("VISA resource name in"=w453, "Gate"=w450, "Drain"=w451, "Timings"=w481, "error in (no error)"=w454, "SMU4"=w441, "sweep mode"=w474, "Panel Controls"=w440) -> ("VG"=w437:dbl[], "Outparams"=w445:T8, "VISA Resource Name out"=w480:refnum<visa-resource-name>, "IS"=w400:dbl[], "ID"=w402:dbl[], "IG"=w399:dbl[], "error out"=w426:errorcluster, "SMU4"=w442:dbl[])  [unwired: 12 in]
        n64 = Unbundle By Name(w445) -> ("V2 Step"=w444:dbl, "V2 Start"=w443:dbl, "Number of points"=w369:i32)
        n65 = Absolute Value(x=w400) -> (abs(x)=w385:dbl[])
        n66 = Absolute Value(x=w402) -> (abs(x)=w401:dbl[])
        n67 = Absolute Value(x=w399) -> (abs(x)=w388:dbl[])
        n68 = Array Size(array=w401) -> (size(s)=w409:i32)
        n69 = Divide(x=w409, y=2) -> (x/y=w352:dbl)
        n70 = Subtract(x=w352, y=1) -> (x-y=w351:dbl)
        n71 = Array Max & Min(array=w385) -> (max value=w392:dbl, min value=w393:dbl)  [unwired: 2 out]
        n72 = Array Max & Min(array=w401) -> (max value=w435:dbl, min value=w398:dbl)  [unwired: 2 out]
        n73 = Array Max & Min(array=w388) -> (max value=w397:dbl, min value=w396:dbl)  [unwired: 2 out]
        n74 = call "4155C Split array.vi"("Number of VAR2 steps"=w369, "Y2 data in"=w402, "X data in"=w437, "Y1 data in"=w400, "Y3 data in"=w399, "error in (no error)"=w426) -> ("Array of clusters"=w428:cluster{"Y data in":dbl[], "X data in":dbl[]}[], "error out"=w357:errorcluster)  [unwired: 1 in]
        n75 = Index Array(array=w385, index=w351) -> (element=w376:dbl)
        n76 = Index Array(array=w385, index=0) -> (element=w377:dbl)
        n77 = Index Array(array=w401, index=w351) -> (element=w378:dbl)
        n78 = Index Array(array=w401, index=0) -> (element=w379:dbl)
        n79 = Index Array(array=w388, index=w351) -> (element=w381:dbl)
        n80 = Index Array(array=w388, index=0) -> (element=w380:dbl)
        n81 = local write "Ig max"(w397) -> ()
        n82 = local write "Ig min"(w396) -> ()
        n83 = local write "Is max"(w392) -> ()
        n84 = local write "Is min"(w393) -> ()
        n85 = local write "Id max"(w435) -> ()
        n86 = local write "Id min"(w398) -> ()
        n87 = local write "I vs Vg"(w428) -> ()
        n88 = Build Array (concatenate)(w391, w392) -> (w370:dbl[])
        n89 = Build Array (concatenate)(w390, w393) -> (w368:dbl[])
        n90 = local write "Is off"(w377) -> ()
        n91 = local write "Is on"(w376) -> ()
        n92 = Build Array (concatenate)(w436, w435) -> (w367:dbl[])
        n93 = Build Array (concatenate)(w423, w398) -> (w366:dbl[])
        n94 = Build Array (concatenate)(w395, w397) -> (w365:dbl[])
        n95 = Build Array (concatenate)(w394, w396) -> (w364:dbl[])
        n96 = Build Array (concatenate)(w383, w376) -> (w363:dbl[])
        n97 = Build Array (concatenate)(w382, w377) -> (w362:dbl[])
        n98 = Build Array (concatenate)(w405, w378) -> (w361:dbl[])
        n99 = Build Array (concatenate)(w406, w379) -> (w360:dbl[])
        n100 = Build Array (concatenate)(w387, w381) -> (w359:dbl[])
        n101 = Build Array (concatenate)(w386, w380) -> (w358:dbl[])
        n102 = local write "Ig off"(w380) -> ()
        n103 = local write "Ig on"(w381) -> ()
        n104 = local write "Id off"(w379) -> ()
        n105 = local write "Id on"(w378) -> ()
        n106 = call "4155C Split array.vi"("Number of VAR2 steps"=w369, "Y2 data in"=w361, "X data in"=w375, "Y1 data in"=w363, "Y3 data in"=w359, "error in (no error)"=w357) -> ("Array of clusters"=w373:cluster{"Y data in":dbl[], "X data in":dbl[]}[], "error out"=w356:errorcluster)  [unwired: 1 in]
        n107 = call "4155C Split array.vi"("Number of VAR2 steps"=w369, "Y2 data in"=w360, "X data in"=w375, "Y1 data in"=w362, "Y3 data in"=w358, "error in (no error)"=w356) -> ("Array of clusters"=w374:cluster{"Y data in":dbl[], "X data in":dbl[]}[], "error out"=w355:errorcluster)  [unwired: 1 in]
        n108 = call "4155C Split array.vi"("Number of VAR2 steps"=w369, "Y2 data in"=w367, "X data in"=w375, "Y1 data in"=w370, "Y3 data in"=w365, "error in (no error)"=w355) -> ("Array of clusters"=w427:cluster{"Y data in":dbl[], "X data in":dbl[]}[], "error out"=w354:errorcluster)  [unwired: 1 in]
        n109 = call "4155C Split array.vi"("Number of VAR2 steps"=w369, "Y2 data in"=w366, "X data in"=w375, "Y1 data in"=w368, "Y3 data in"=w364, "error in (no error)"=w354) -> ("Array of clusters"=w424:cluster{"Y data in":dbl[], "X data in":dbl[]}[], "error out"=w353:errorcluster)  [unwired: 1 in]
        n110 = Open/Create/Replace File(file path (use dialog)=w484, error in=w353, operation (0:open)=w438) -> (refnum out=w421:refnum<file>, error out=w419:errorcluster)  [unwired: 3 in, 1 out]
        n111 = call "4155C Make Big 2d array.vi"("1D Var1"=w437, "1d IS"=w400, "1d ID"=w402, "1d IG"=w399, "1d SMU4"=w442, "SMU4"=w441, "VAR2 START"=w443, "Number of VAR2 steps"=w369, "VAR2 STEP"=w444, "VAR1 Name"="Vg", "Decimal places in header"=i8 1, "VAR2 Name"="Vd") -> ("Header array"=w422:string[], "Data array"=w420:dbl[][])  [unwired: 14 in]
        n112 = local write "Imax vs time"(w427) -> ()
        n113 = local write "Imin vs time"(w424) -> ()
        n114 = local write "Ion vs time"(w373) -> ()
        n115 = local write "Ioff vs time"(w374) -> ()
        n116 = call "4155C Config Chart Colours.vi"("Numeric"=w369, "XY Graph 2"=w404) -> ()  [unwired: 6 in]
        n117 = call "4155C Config Chart Colours.vi"("Numeric"=w369, "XY Graph 2"=w403) -> ()  [unwired: 6 in]
        n118 = call "4155C Config Chart Colours.vi"("Numeric"=w369, "XY Graph 2"=w372) -> ()  [unwired: 6 in]
        n119 = call "4155C Config Chart Colours.vi"("Numeric"=w369, "XY Graph 2"=w371) -> ()  [unwired: 6 in]
        n120 = call "4155C Config Chart Colours.vi"("Numeric"=w369, "XY Graph 2"=w434) -> ()  [unwired: 6 in]
        n121 = call "4155C Write array to file.vi"("Byte Stream File Refnum"=w421, "Header"=w422, "Data Array"=w420, "error in (no error)"=w419) -> ("dup refnum"=w418:refnum<file>, "error out"=w417:errorcluster)  [unwired: 1 in]
        n122 = Close File(refnum=w418, error in=w417) -> (error out=w479:errorcluster)  [unwired: 1 out]
      }
      frame "pulsedstressV" {
        w521 = 0
        n123 = Number To Decimal String(number=w512) -> (decimal integer string=w568:string)  [unwired: 1 in]
        n124 = Delete From Array(array=w502, index=0 ("Index")) -> (deleted portion=w559:string, array with subset deleted=w558:string[])  [unwired: 1 in]
        n125 = Bundle By Name(cluster=w538, "Emergency Stop"=w571) -> (w540:T2)
        n126 = VISA Write(VISA resource name=w552, write buffer=":PAGE:CHAN:MODE SWE;" ("write buffer (\"\")"), error in (no error)=w551) -> (VISA resource name out=w549:refnum<visa-resource-name>, error out=w550:errorcluster)  [unwired: 1 out]
        n127 = Concatenate Strings(w567, "-pulsedstressV-" ("Substring"), w568, w511, ".txt" ("Substring")) -> (w570:string)
        n128 = case shown="\"d\", Default" w559 {
          tunnel: [w580 w581] -> w557
          frame "s" {
            w580 = u16 0 items=["Single", "Double"] ("sweep mode")
          }
          frame "d", Default {
            w581 = u16 1 items=["Single", "Double"] ("sweep mode")
          }
        }
        n129 = Fract/Exp String To Number(string=w558) -> (number=w553:dbl[])  [unwired: 3 in, 1 out]
        n130 = String To Path(string=w570) -> (path=w566:path)
        n131 = Index Array(array=w553, index #1=0 ("Index")) -> (element #1=w530:dbl, element #2=w529:dbl, element #3=w526:dbl, element #4=w525:dbl, element #5=w524:dbl, element #6=w528:dbl)  [unwired: 5 in]
        n132 = Bundle By Name(cluster=w527, "Pulse period"=w525, "Base voltage"=w526, "Pulse width"=w524) -> (w523:T6)
        n133 = Unbundle By Name(w523) -> ("Pulse period"=w531:dbl)
        n134 = Bundle By Name(cluster=w555, "Gate Start"=w529, "Gate Stop"=w530, "Gate Step (linear only)"=0, "Gate Compliance"=w564, "Range mode"=w545, "Range"=w544) -> (w546:T4)
        n135 = call <vilib>:"compatOverwrite.vi"("overwrite (F)"=TRUE) -> ("overwrite?"=w516:T7)
        n136 = Bundle By Name(cluster=w554, "Drain Start"=w528, "Drain Stop"=w521, "Drain Step"=w521, "Drain Compliance"=w565, "Range mode"=w543, "Range"=w542) -> (w547:T5)
        n137 = call "4155C PulsedStressV.vi"("VISA resource name in"=w549, "sweep mode"=w557, "Panel Controls"=w540, "Gate"=w546, "Drain"=w547, "Timings"=w523, "error in (no error)"=w550, "SMU4"=w539) -> ("VISA Resource Name out"=w562:refnum<visa-resource-name>, "ID"=w519:dbl[], "IG"=w517:dbl[], "Outparams"=w541:T8, "error out"=w563:errorcluster)  [unwired: 3 in]
        n138 = Unbundle By Name(w541) -> ("Number of points"=w518:i32)  [unwired: 2 out]
        n139 = for {
          N: w518 -> [_]
          tunnel: [w577] -> w520 mode=indexing
          tunnel: w531 -> [w579]
          i -> [w578]
          n140 = Multiply(x=w579, y=w578) -> (x*y=w577:dbl)
        }
        n141 = Insert Into Array(array=dbl[][] [] ("Input Array"), new element=w520) -> (w532:dbl[][])  [unwired: 2 in]
        n142 = Insert Into Array(array=w532, new element=w519) -> (w537:dbl[][])  [unwired: 2 in]
        n143 = Insert Into Array(array=w537, new element=w517) -> (w536:dbl[][])  [unwired: 2 in]
        n144 = Transpose 2D Array(2D array=w536) -> (transposed array=w535:dbl[][])
        n145 = Open/Create/Replace File(file path (use dialog)=w566, error in=w563, operation (0:open)=w516) -> (refnum out=w574:refnum<file>, error out=w575:errorcluster)  [unwired: 3 in, 1 out]
        n146 = call "4155C Write array to file.vi"("Byte Stream File Refnum"=w574, "Header"=string[] ["Time /s", "Id /A", "Ig /A"], "Data Array"=w535, "error in (no error)"=w575) -> ("dup refnum"=w572:refnum<file>, "error out"=w573:errorcluster)  [unwired: 1 in]
        n147 = Close File(refnum=w572, error in=w573) -> (error out=w561:errorcluster)  [unwired: 1 out]
      }
      frame "transfer-fpp" {
        n148 = Number To Decimal String(number=w603) -> (decimal integer string=w657:string)  [unwired: 1 in]
        n149 = Bundle By Name(cluster=w633, "Emergency Stop"=w661) -> (w669:T1)
        n150 = Delete From Array(array=w648, index=0 ("Index")) -> (deleted portion=w646:string, array with subset deleted=w645:string[])  [unwired: 1 in]
        n151 = Concatenate Strings(w656, "-transferfpp-" ("Substring"), w657, w601, ".txt" ("Substring")) -> (w659:string)
        n152 = VISA Write(VISA resource name=w625, write buffer=":PAGE:CHAN:MODE SWE;" ("write buffer (\"\")"), error in (no error)=w624) -> (VISA resource name out=w622:refnum<visa-resource-name>, error out=w623:errorcluster)  [unwired: 1 out]
        n153 = case shown="\"d\", Default" w646 {
          tunnel: [w670 w671] -> w644
          frame "s" {
            w670 = u16 0 items=["Single", "Double"] ("sweep mode")
          }
          frame "d", Default {
            w671 = u16 1 items=["Single", "Double"] ("sweep mode")
          }
        }
        n154 = Fract/Exp String To Number(string=w645) -> (number=w629:dbl[])  [unwired: 3 in, 1 out]
        n155 = String To Path(string=w659) -> (path=w655:path)
        n156 = Index Array(array=w629, index #1=0 ("Index")) -> (element #1=w643:dbl, element #2=w642:dbl, element #3=w641:dbl)  [unwired: 2 in]
        n157 = Delete From Array(array=w629, length=3 ("Length"), index=0 ("Index")) -> (array with subset deleted=w627:dbl[])  [unwired: 1 out]
        n158 = Bundle By Name(cluster=w635, "Gate Start"=w643, "Gate Stop"=w642, "Gate Step (linear only)"=w641, "Gate Compliance"=w653, "Range mode"=w618, "Range"=w617) -> (w619:T4)
        n159 = Index Array(array=w627, index #1=0 ("Index")) -> (element #1=w638:dbl, element #2=w637:dbl, element #3=w636:dbl)  [unwired: 2 in]
        n160 = call <vilib>:"compatOverwrite.vi"("overwrite (F)"=TRUE) -> ("overwrite?"=w606:T7)
        n161 = Bundle By Name(cluster=w634, "Drain Start"=w638, "Drain Stop"=w637, "Drain Step"=w636, "Drain Compliance"=w654, "Range mode"=w616, "Range"=w615) -> (w620:T5)
        n162 = call "4155C Transfer-FPP.vi"("VISA resource name in"=w622, "Gate"=w619, "Drain"=w620, "Timings"=w652, "error in (no error)"=w623, "sweep mode"=w644, "Panel Controls"=w669) -> ("VG"=w660:dbl[], "Outparams"=w614:T8, "VISA Resource Name out"=w650:refnum<visa-resource-name>, "Vprobe2"=w610:dbl[], "ID"=w609:dbl[], "IG"=w608:dbl[], "Vprobe1"=w607:dbl[], "error out"=w651:errorcluster)  [unwired: 13 in]
        n163 = Unbundle By Name(w614) -> ("V2 Step"=w613:dbl, "V2 Start"=w612:dbl, "Number of points"=w611:i32)
        n164 = Open/Create/Replace File(file path (use dialog)=w655, error in=w651, operation (0:open)=w606) -> (refnum out=w666:refnum<file>, error out=w667:errorcluster)  [unwired: 3 in, 1 out]
        n165 = call "4155C Make Big 2d array FPP.vi"("1D Var1"=w660, "1d ID"=w609, "1d Vp2"=w610, "1d IG"=w608, "1d Vp1"=w607, "VAR2 START"=w612, "Number of VAR2 steps"=w611, "VAR2 STEP"=w613, "VAR1 Name"="Vg", "Decimal places in header"=i8 1, "VAR2 Name"="Vd") -> ("Header array"=w662:string[], "Data array"=w663:dbl[][])  [unwired: 15 in]
        n166 = call "4155C Write array to file.vi"("Byte Stream File Refnum"=w666, "Header"=w662, "Data Array"=w663, "error in (no error)"=w667) -> ("dup refnum"=w664:refnum<file>, "error out"=w665:errorcluster)  [unwired: 1 in]
        n167 = Close File(refnum=w664, error in=w665) -> (error out=w649:errorcluster)  [unwired: 1 out]
      }
      frame "output" {
        n168 = Number To Decimal String(number=w701) -> (decimal integer string=w750:string)  [unwired: 1 in]
        n169 = Bundle By Name(cluster=w727, "Emergency Stop"=w752) -> (w762:T1)
        n170 = Delete From Array(array=w742, index=0 ("Index")) -> (deleted portion=w740:string, array with subset deleted=w739:string[])  [unwired: 1 in]
        n171 = Concatenate Strings(w749, w672, w750, w700, "_O.txt" ("Suffix (output)")) -> (w751:string)
        n172 = VISA Write(VISA resource name=w718, write buffer=":PAGE:CHAN:MODE SWE;" ("write buffer (\"\")"), error in (no error)=w715) -> (VISA resource name out=w717:refnum<visa-resource-name>, error out=w716:errorcluster)  [unwired: 1 out]
        n173 = case shown="\"d\", Default" w740 {
          tunnel: [w763 w764] -> w738
          frame "s" {
            w763 = u16 0 items=["Single", "Double"] ("sweep mode")
          }
          frame "d", Default {
            w764 = u16 1 items=["Single", "Double"] ("sweep mode")
          }
        }
        n174 = Fract/Exp String To Number(string=w739) -> (number=w721:dbl[])  [unwired: 3 in, 1 out]
        n175 = String To Path(string=w751) -> (path=w748:path)
        n176 = Index Array(array=w721, index #1=0 ("Index")) -> (element #1=w737:dbl, element #2=w736:dbl, element #3=w735:dbl)  [unwired: 2 in]
        n177 = Delete From Array(array=w721, length=3 ("Length"), index=0 ("Index")) -> (array with subset deleted=w720:dbl[])  [unwired: 1 out]
        n178 = control-ref of="I vs Vd"() -> (w691:refnum<vi>)
        n179 = Bundle By Name(cluster=w729, "Gate Start"=w737, "Gate Stop"=w736, "Gate Step (linear only)"=w735, "Gate Compliance"=w746, "Range mode"=w713, "Range"=w712) -> (w761:T4)
        n180 = Index Array(array=w720, index #1=0 ("Index")) -> (element #1=w732:dbl, element #2=w731:dbl, element #3=w730:dbl)  [unwired: 2 in]
        n181 = call <vilib>:"compatOverwrite.vi"("overwrite (F)"=TRUE) -> ("overwrite?"=w705:T7)
        n182 = Bundle By Name(cluster=w728, "Drain Start"=w732, "Drain Stop"=w731, "Drain Step"=w730, "Drain Compliance"=w747, "Range mode"=w711, "Range"=w714) -> (w760:T5)
        n183 = call "4155C Output.vi"("VISA resource name in"=w717, "Gate"=w761, "Drain"=w760, "Timings"=w745, "error in (no error)"=w716, "SMU4"=w707, "sweep mode"=w738, "Panel controls"=w762) -> ("VD"=w698:dbl[], "Outparams"=w709:T8, "VISA Resource Name out"=w744:refnum<visa-resource-name>, "IS"=w697:dbl[], "ID"=w696:dbl[], "IG"=w695:dbl[], "error out"=w693:errorcluster, "SMU4"=w706:dbl[])  [unwired: 12 in]
        n184 = Unbundle By Name(w709) -> ("V2 Step"=w710:dbl, "V2 Start"=w708:dbl, "Number of points"=w690:i32)
        n185 = call "4155C Split array.vi"("Number of VAR2 steps"=w690, "Y2 data in"=w696, "X data in"=w698, "Y1 data in"=w697, "Y3 data in"=w695, "error in (no error)"=w693) -> ("Array of clusters"=w694:cluster{"Y data in":dbl[], "X data in":dbl[]}[], "error out"=w692:errorcluster)  [unwired: 1 in]
        n186 = local write "I vs Vd"(w694) -> ()
        n187 = call "4155C Config Chart Colours.vi"("Numeric"=w690, "XY Graph 2"=w691) -> ()  [unwired: 6 in]
        n188 = Open/Create/Replace File(file path (use dialog)=w748, error in=w692, operation (0:open)=w705) -> (refnum out=w757:refnum<file>, error out=w758:errorcluster)  [unwired: 3 in, 1 out]
        n189 = call "4155C Make Big 2d array.vi"("1D Var1"=w698, "1d IS"=w697, "1d ID"=w696, "1d IG"=w695, "1d SMU4"=w706, "SMU4"=w707, "VAR2 START"=w708, "Number of VAR2 steps"=w690, "VAR2 STEP"=w710, "VAR1 Name"="Vd", "Decimal places in header"=i8 1, "VAR2 Name"="Vg") -> ("Header array"=w753:string[], "Data array"=w754:dbl[][])  [unwired: 14 in]
        n190 = call "4155C Write array to file.vi"("Byte Stream File Refnum"=w757, "Header"=w753, "Data Array"=w754, "error in (no error)"=w758) -> ("dup refnum"=w755:refnum<file>, "error out"=w756:errorcluster)  [unwired: 1 in]
        n191 = Close File(refnum=w755, error in=w756) -> (error out=w743:errorcluster)  [unwired: 1 out]
      }
      frame "output-fpp" {
        n192 = Number To Decimal String(number=w785) -> (decimal integer string=w839:string)  [unwired: 1 in]
        n193 = Bundle By Name(cluster=w815, "Emergency Stop"=w842) -> (w852:T1)
        n194 = Delete From Array(array=w830, index=0 ("Index")) -> (deleted portion=w828:string, array with subset deleted=w827:string[])  [unwired: 1 in]
        n195 = VISA Write(VISA resource name=w806, write buffer=":PAGE:CHAN:MODE SWE;" ("write buffer (\"\")"), error in (no error)=w803) -> (VISA resource name out=w805:refnum<visa-resource-name>, error out=w804:errorcluster)  [unwired: 1 out]
        n196 = Concatenate Strings(w838, "-outputfpp-" ("Substring"), w839, w784, ".txt" ("Substring")) -> (w841:string)
        n197 = case shown="\"d\", Default" w828 {
          tunnel: [w853 w854] -> w826
          frame "s" {
            w853 = u16 0 items=["Single", "Double"] ("sweep mode")
          }
          frame "d", Default {
            w854 = u16 1 items=["Single", "Double"] ("sweep mode")
          }
        }
        n198 = Fract/Exp String To Number(string=w827) -> (number=w809:dbl[])  [unwired: 3 in, 1 out]
        n199 = String To Path(string=w841) -> (path=w837:path)
        n200 = Index Array(array=w809, index #1=0 ("Index")) -> (element #1=w825:dbl, element #2=w824:dbl, element #3=w823:dbl)  [unwired: 2 in]
        n201 = Delete From Array(array=w809, length=3 ("Length"), index=0 ("Index")) -> (array with subset deleted=w808:dbl[])  [unwired: 1 out]
        n202 = Bundle By Name(cluster=w817, "Gate Start"=w825, "Gate Stop"=w824, "Gate Step (linear only)"=w823, "Gate Compliance"=w835, "Range mode"=w801, "Range"=w800) -> (w851:T4)
        n203 = Index Array(array=w808, index #1=0 ("Index")) -> (element #1=w820:dbl, element #2=w819:dbl, element #3=w818:dbl)  [unwired: 2 in]
        n204 = call <vilib>:"compatOverwrite.vi"("overwrite (F)"=TRUE) -> ("overwrite?"=w789:T7)
        n205 = Bundle By Name(cluster=w816, "Drain Start"=w820, "Drain Stop"=w819, "Drain Step"=w818, "Drain Compliance"=w836, "Range mode"=w799, "Range"=w802) -> (w850:T5)
        n206 = call "4155C Output-FPP.vi"("VISA resource name in"=w805, "Gate"=w851, "Drain"=w850, "Timings"=w834, "error in (no error)"=w804, "sweep mode"=w826, "Panel controls"=w852) -> ("VD"=w794:dbl[], "Outparams"=w797:T8, "VISA Resource Name out"=w832:refnum<visa-resource-name>, "Vprobe2"=w793:dbl[], "ID"=w792:dbl[], "IG"=w791:dbl[], "Vprobe1"=w790:dbl[], "error out"=w833:errorcluster)  [unwired: 13 in]
        n207 = Unbundle By Name(w797) -> ("V2 Step"=w798:dbl, "V2 Start"=w796:dbl, "Number of points"=w795:i32)
        n208 = Open/Create/Replace File(file path (use dialog)=w837, error in=w833, operation (0:open)=w789) -> (refnum out=w847:refnum<file>, error out=w848:errorcluster)  [unwired: 3 in, 1 out]
        n209 = call "4155C Make Big 2d array FPP.vi"("1D Var1"=w794, "1d ID"=w792, "1d Vp2"=w793, "1d IG"=w791, "1d Vp1"=w790, "VAR2 START"=w796, "Number of VAR2 steps"=w795, "VAR2 STEP"=w798, "VAR1 Name"="Vd", "Decimal places in header"=i8 1, "VAR2 Name"="Vg") -> ("Header array"=w843:string[], "Data array"=w844:dbl[][])  [unwired: 15 in]
        n210 = call "4155C Write array to file.vi"("Byte Stream File Refnum"=w847, "Header"=w843, "Data Array"=w844, "error in (no error)"=w848) -> ("dup refnum"=w845:refnum<file>, "error out"=w846:errorcluster)  [unwired: 1 in]
        n211 = Close File(refnum=w845, error in=w846) -> (error out=w831:errorcluster)  [unwired: 1 out]
      }
      frame "itime" {
        n212 = Delete From Array(array=w887, index=0 ("Index")) -> (deleted portion=w888:string)  [unwired: 1 in, 1 out]
        n213 = case shown="\"s\"" w888 {
          tunnel: w886 -> [w892 w894 w897]
          tunnel: [w891 w893 w896] -> w879
          frame "s" {
            w890 = u32 0 items=["short  ", "medium  ", "long  "] ("integration time 2")
            n214 = Bundle By Name(cluster=w892, "integration time"=w890) -> (w891:T6)
          }
          frame "m", Default {
            w895 = u32 1 items=["short  ", "medium  ", "long  "] ("integration time 2")
            n215 = Bundle By Name(cluster=w894, "integration time"=w895) -> (w893:T6)
          }
          frame "l" {
            w898 = u32 2 items=["short  ", "medium  ", "long  "] ("integration time 2")
            n216 = Bundle By Name(cluster=w897, "integration time"=w898) -> (w896:T6)
          }
        }
      }
      frame "pulsed" {
        n217 = Delete From Array(array=w932, index=0 ("Index")) -> (deleted portion=w933:string, array with subset deleted=w920:string[])  [unwired: 1 in]
        n218 = case shown="\"on\", Default" w933 {
          tunnel: w931 -> [w943 w946]
          tunnel: [w942 w945] -> w924
          tunnel: w920 -> [w940 _]
          frame "on", Default {
            w941 = u16 1 items=["Continuous", "Pulsed"] ("sweep method")
            n219 = Fract/Exp String To Number(string=w940) -> (number=w938:dbl[])  [unwired: 3 in, 1 out]
            n220 = Index Array(array=w938, index #1=0 ("Index")) -> (element #1=w937:dbl, element #2=w936:dbl, element #3=w935:dbl)  [unwired: 2 in]
            n221 = Bundle By Name(cluster=w943, "sweep method"=w941, "Pulse period"=w937, "Base voltage"=w936, "Pulse width"=w935) -> (w942:T6)
          }
          frame "off" {
            w944 = u16 0 items=["Continuous", "Pulsed"] ("sweep method")
            n222 = Bundle By Name(cluster=w946, "sweep method"=w944) -> (w945:T6)
          }
        }
      }
      frame "gaterangemode" {
        n223 = Delete From Array(array=w978, index=0 ("Index")) -> (deleted portion=w979:string)  [unwired: 1 in, 1 out]
        n224 = case shown="\"f\"" w979 {
          tunnel: [w981 w982 w983] -> w968
          frame "a", Default {
            w981 = u16 0 items=["Auto", "Limited", "Fixed"] ("Gate Range\nmode 2")
          }
          frame "f" {
            w982 = u16 2 items=["Auto", "Limited", "Fixed"] ("Gate Range\nmode 2")
          }
          frame "l" {
            w983 = u16 1 items=["Auto", "Limited", "Fixed"] ("Gate Range\nmode 2")
          }
        }
      }
      frame "gaterange" {
        (unwired) u8 11 items=["10fA  ", "100fA  ", "1nA  ", "10nA", "100nA", "1uA", "10uA", "100uA", "1mA", "10mA", "100mA", "1A"] ("Gate Range 2")
        n225 = Delete From Array(array=w1022, index=0 ("Index")) -> (deleted portion=w1012:string)  [unwired: 1 in, 1 out]
        n226 = Scan Value(string=w1012, format string="") -> (value=w1010:dbl)  [unwired: 1 in, 1 out]
        n227 = Logarithm Base 10(1:w1010) -> (0:w1009:dbl)
        n228 = Round To Nearest(number=w1009) -> (nearest integer value=w1008:dbl)
        n229 = Add(x=w1008, y=11.0) -> (x+y=w1006:dbl)
        n230 = To Unsigned Byte Integer(number=w1006) -> (unsigned 8bit integer=w1005:u8)
      }
      frame "drainrange" {
        (unwired) u8 11 items=["10fA  ", "100fA  ", "1nA  ", "10nA", "100nA", "1uA", "10uA", "100uA", "1mA", "10mA", "100mA", "1A"] ("Gate Range 2")
        n231 = Delete From Array(array=w1062, index=0 ("Index")) -> (deleted portion=w1053:string)  [unwired: 1 in, 1 out]
        n232 = Scan Value(string=w1053, format string="") -> (value=w1051:dbl)  [unwired: 1 in, 1 out]
        n233 = Logarithm Base 10(1:w1051) -> (0:w1050:dbl)
        n234 = Round To Nearest(number=w1050) -> (nearest integer value=w1049:dbl)
        n235 = Add(x=w1049, y=11.0) -> (x+y=w1047:dbl)
        n236 = To Unsigned Byte Integer(number=w1047) -> (unsigned 8bit integer=w1046:u8)
      }
      frame "drainrangemode" {
        n237 = Delete From Array(array=w1095, index=0 ("Index")) -> (deleted portion=w1096:string)  [unwired: 1 in, 1 out]
        n238 = case shown="\"f\"" w1096 {
          tunnel: [w1098 w1099 w1100] -> w1085
          frame "a", Default {
            w1098 = u16 0 items=["Auto", "Limited", "Fixed"] ("Gate Range\nmode 2")
          }
          frame "f" {
            w1099 = u16 2 items=["Auto", "Limited", "Fixed"] ("Gate Range\nmode 2")
          }
          frame "l" {
            w1100 = u16 1 items=["Auto", "Limited", "Fixed"] ("Gate Range\nmode 2")
          }
        }
      }
      frame "Error", Default {
      }
      frame "logfile" {
        n239 = Number To Decimal String(number=w1153) -> (decimal integer string=w1188:string)  [unwired: 1 in]
        n240 = Concatenate Strings(w1187, "logfile" ("Substring"), w1188, w1151, ".txt" ("Substring")) -> (w1185:string)
        n241 = String To Path(string=w1185) -> (path=w1158:path)
        n242 = Unbundle(w1184) -> ("integration time"=w1183:u32, "Short/Long integration time"=w1182:dbl, "hold time (sec)"=w1181:dbl, "delay time (sec)"=w1180:dbl, "Step Time (0 disables)"=w1179:dbl, "sweep method"=w1178:u16, "Pulse period"=w1177:dbl, "Base voltage"=w1176:dbl, "Pulse width"=w1175:dbl)
        n243 = Build Array(w1183, w1182, w1181, w1180, w1179, w1178, w1177, w1176, w1175, w1169, w1170, w1171, w1172, w1173, w1174) -> (w1162:dbl[])
        n244 = Insert Into Array(array=dbl[][] [] ("Input Array"), new element=w1162) -> (w1161:dbl[][])  [unwired: 2 in]
        n245 = call <vilib>:"compatOverwrite.vi"("overwrite (F)"=TRUE) -> ("overwrite?"=w1156:T7)
        n246 = Open/Create/Replace File(file path (use dialog)=w1158, error in=w1160, operation (0:open)=w1156) -> (refnum out=w1166:refnum<file>, error out=w1165:errorcluster)  [unwired: 3 in, 1 out]
        n247 = call "4155C Write array to file.vi"("Byte Stream File Refnum"=w1166, "Header"=string[] ["Int Time", "Short/Long Itime", "Hold time", "Delay time", "Step time", "Sweep method", "Pulse period", "Base Voltage", "Pulse width", "Drain compliance", "Gate compliance", "Gate range mode", "Gate range", "S/D range mode", "S/D range"], "Data Array"=w1161, "error in (no error)"=w1165) -> ("dup refnum"=w1168:refnum<file>, "error out"=w1167:errorcluster)  [unwired: 1 in]
        n248 = Close File(refnum=w1168, error in=w1167) -> (error out=w1159:errorcluster)  [unwired: 1 out]
      }
      frame "sample" {
        n249 = Number To Decimal String(number=w1211) -> (decimal integer string=w1259:string)  [unwired: 1 in]
        n250 = Fract/Exp String To Number(string=w1256) -> (number=w1217:dbl[])  [unwired: 3 in, 1 out]
        n251 = Concatenate Strings(w1234, "-sample-" ("Substring"), w1259, w1209, ".txt" ("Substring")) -> (w1257:string)
        n252 = Index Array(array=w1217, index=0 ("Index")) -> (element=w1254:dbl)
        n253 = String To Path(string=w1257) -> (path=w1238:path)
        n254 = Index Array(array=w1217, index=2 ("Index")) -> (element=w1250:dbl)
        n255 = Index Array(array=w1217, index=3 ("Index")) -> (element=w1219:dbl)
        n256 = Index Array(array=w1217, index=4 ("Index")) -> (element=w1216:dbl)
        n257 = call "4155C Config Sampling Measurements.vi"("Sampling interval"=w1216, "Sample time"=w1219, "Display on/off"=TRUE, "Timings"=w1225, "Num Points"=w1250, "error in (no error)"=w1261, "Drain Compliance"=w1260, "Gate Compliance"=w1235, "VISA session"=w1262) -> ("error out"=w1263:errorcluster, "dup VISA resource name"=w1264:refnum<visa-resource-name>)  [unwired: 1 in]
        n258 = Index Array(array=w1217, index=1 ("Index")) -> (element=w1251:dbl)
        n259 = call "4155C Take Sample.vi"("Emergency Stop"=w1231, "error in (no error)"=w1263, "Vd"=w1251, "Vg"=w1254, "VISA resource name in"=w1264) -> ("error out"=w1229:errorcluster, "Id"=w1266:dbl[], "Ig"=w1240:dbl[], "VISA Resource Name out"=w1227:refnum<visa-resource-name>, "Is"=w1265:dbl[], "Time"=w1244:dbl[])  [unwired: 1 in]
        n260 = Insert Into Array(array=dbl[][] [] ("Input Array"), new element=w1244) -> (w1243:dbl[][])  [unwired: 2 in]
        n261 = Insert Into Array(array=w1243, new element=w1240) -> (w1242:dbl[][])  [unwired: 2 in]
        n262 = Insert Into Array(array=w1242, new element=w1266) -> (w1241:dbl[][])  [unwired: 2 in]
        n263 = VISA Write(VISA resource name=w1227, write buffer=":DISP ON" ("write buffer (\"\")"), error in (no error)=w1229) -> (VISA resource name out=w1226:refnum<visa-resource-name>, error out=w1228:errorcluster)  [unwired: 1 out]
        n264 = Insert Into Array(array=w1241, new element=w1265) -> (w1233:dbl[][])  [unwired: 2 in]
        n265 = Transpose 2D Array(2D array=w1233) -> (transposed array=w1232:dbl[][])
        n266 = call <vilib>:"compatOverwrite.vi"("overwrite (F)"=TRUE) -> ("overwrite?"=w1214:T7)
        n267 = Open/Create/Replace File(file path (use dialog)=w1238, error in=w1228, operation (0:open)=w1214) -> (refnum out=w1247:refnum<file>, error out=w1246:errorcluster)  [unwired: 3 in, 1 out]
        n268 = call "4155C Write array to file.vi"("Byte Stream File Refnum"=w1247, "Header"=string[] ["Time /s", "Ig /A", "Id /A", "Is /A"], "Data Array"=w1232, "error in (no error)"=w1246) -> ("dup refnum"=w1249:refnum<file>, "error out"=w1248:errorcluster)  [unwired: 1 in]
        n269 = Close File(refnum=w1249, error in=w1248) -> (error out=w1236:errorcluster)  [unwired: 1 out]
      }
      frame "samplei" {
        n270 = Number To Decimal String(number=w1288) -> (decimal integer string=w1339:string)  [unwired: 1 in]
        n271 = Concatenate Strings(w1318, "-samplei-" ("Substring"), w1339, w1287, ".txt" ("Substring")) -> (w1337:string)
        n272 = Fract/Exp String To Number(string=w1336) -> (number=w1303:dbl[])  [unwired: 3 in, 1 out]
        n273 = String To Path(string=w1337) -> (path=w1321:path)
        n274 = Index Array(array=w1303, index=4 ("Index")) -> (element=w1297:dbl)
        n275 = Index Array(array=w1303, index=3 ("Index")) -> (element=w1298:dbl)
        n276 = Index Array(array=w1303, index=1 ("Index")) -> (element=w1300:dbl)
        n277 = Index Array(array=w1303, index=0 ("Index")) -> (element=w1301:dbl)
        n278 = Index Array(array=w1303, index=2 ("Index")) -> (element=w1299:dbl)
        n279 = call "4155C Config SamplingI Measurements.vi"("Sample time"=w1299, "Display on/off"=TRUE, "Timings"=w1310, "Num Points"=w1300, "error in (no error)"=w1341, "Sampling interval"=w1298, "VISA session"=w1342) -> ("error out"=w1343:errorcluster, "dup VISA resource name"=w1344:refnum<visa-resource-name>)  [unwired: 3 in]
        n280 = call "4155C Take SampleI.vi"("Emergency Stop"=w1315, "error in (no error)"=w1343, "Idg 2"=w1301, "Vdg compliance 2"=w1297, "VISA resource name in"=w1344) -> ("error out"=w1313:errorcluster, "Idg"=w1346:dbl[], "Vdg"=w1323:dbl[], "VISA Resource Name out"=w1311:refnum<visa-resource-name>, "Is"=w1345:dbl[], "Time"=w1327:dbl[])  [unwired: 1 in]
        n281 = Insert Into Array(array=dbl[][] [] ("Input Array"), new element=w1327) -> (w1326:dbl[][])  [unwired: 2 in]
        n282 = Insert Into Array(array=w1326, new element=w1323) -> (w1325:dbl[][])  [unwired: 2 in]
        n283 = Insert Into Array(array=w1325, new element=w1346) -> (w1324:dbl[][])  [unwired: 2 in]
        n284 = VISA Write(VISA resource name=w1311, write buffer=":DISP ON" ("write buffer (\"\")"), error in (no error)=w1313) -> (VISA resource name out=w1296:refnum<visa-resource-name>, error out=w1312:errorcluster)  [unwired: 1 out]
        n285 = Insert Into Array(array=w1324, new element=w1345) -> (w1317:dbl[][])  [unwired: 2 in]
        n286 = call <vilib>:"compatOverwrite.vi"("overwrite (F)"=TRUE) -> ("overwrite?"=w1291:T7)
        n287 = Open/Create/Replace File(file path (use dialog)=w1321, error in=w1312, operation (0:open)=w1291) -> (refnum out=w1330:refnum<file>, error out=w1329:errorcluster)  [unwired: 3 in, 1 out]
        n288 = Transpose 2D Array(2D array=w1317) -> (transposed array=w1316:dbl[][])
        n289 = call "4155C Write array to file.vi"("Byte Stream File Refnum"=w1330, "Header"=string[] ["Time /s", "Vdg /V", "Idg /A", "Is /A"], "Data Array"=w1316, "error in (no error)"=w1329) -> ("dup refnum"=w1332:refnum<file>, "error out"=w1331:errorcluster)  [unwired: 1 in]
        n290 = Close File(refnum=w1332, error in=w1331) -> (error out=w1294:errorcluster)  [unwired: 1 out]
        n291 = VISA Write(VISA resource name=w1296, write buffer=";:PAGE:SCON:STAN OFF;:PAGE:CHAN:VSU2:DIS;" ("write buffer (\"\")"), error in (no error)=w1294) -> (VISA resource name out=w1292:refnum<visa-resource-name>, error out=w1293:errorcluster)  [unwired: 1 out]
      }
      frame "#" {
        n292 = VISA Write(VISA resource name=w1372, write buffer=":DISP ON" ("write buffer (\"\")"), error in (no error)=w1371) -> (VISA resource name out=w1370:refnum<visa-resource-name>, error out=w1369:errorcluster)  [unwired: 1 out]
      }
      frame "stressV" {
        n293 = Number To Decimal String(number=w1401) -> (decimal integer string=w1442:string)  [unwired: 1 in]
        n294 = Concatenate Strings(w1426, "-stressV-" ("Substring"), w1442, w1400, ".txt" ("Substring")) -> (w1440:string)
        n295 = Fract/Exp String To Number(string=w1439) -> (number=w1412:dbl[])  [unwired: 3 in, 1 out]
        n296 = String To Path(string=w1440) -> (path=w1430:path)
        n297 = Index Array(array=w1412, index=3 ("Index")) -> (element=w1409:dbl)
        n298 = Index Array(array=w1412, index=1 ("Index")) -> (element=w1407:dbl)
        n299 = Index Array(array=w1412, index=0 ("Index")) -> (element=w1406:dbl)
        n300 = Index Array(array=w1412, index=4 ("Index")) -> (element=w1411:dbl)
        n301 = Index Array(array=w1412, index=2 ("Index")) -> (element=w1408:dbl)
        n302 = call "4155C Config V Stress.vi"("VISA session"=w1445, "ID compliance"=w1409, "VD"=w1407, "VG"=w1406, "IG compliance"=w1408, "error in (no error)"=w1444, "Display on/off"=TRUE) -> ("dup VISA resource name"=w1447:refnum<visa-resource-name>, "error out"=w1446:errorcluster)
        n303 = call "4155C Apply Stress.vi"("error in (no error)"=w1446, "Duration"=w1411, "Emergency Stop"=w1425, "VISA resource name in"=w1447) -> ("error out"=w1423:errorcluster, "VISA Resource Name out"=w1421:refnum<visa-resource-name>)
        n304 = VISA Write(VISA resource name=w1421, write buffer=":DISP ON" ("write buffer (\"\")"), error in (no error)=w1423) -> (VISA resource name out=w1420:refnum<visa-resource-name>, error out=w1422:errorcluster)  [unwired: 1 out]
        n305 = call <vilib>:"compatOverwrite.vi"("overwrite (F)"=TRUE) -> ("overwrite?"=w1405:T7)
        n306 = Open/Create/Replace File(file path (use dialog)=w1430, error in=w1422, operation (0:open)=w1405) -> (refnum out=w1433:refnum<file>, error out=w1432:errorcluster)  [unwired: 3 in, 1 out]
        n307 = call "4155C Write array to file.vi"("Byte Stream File Refnum"=w1433, "Header"=string[] ["V stress completed successfully", ""], "error in (no error)"=w1432) -> ("dup refnum"=w1435:refnum<file>, "error out"=w1434:errorcluster)  [unwired: 2 in]
        n308 = Close File(refnum=w1435, error in=w1434) -> (error out=w1428:errorcluster)  [unwired: 1 out]
      }
      frame "stressI" {
        n309 = Number To Decimal String(number=w1468) -> (decimal integer string=w1505:string)  [unwired: 1 in]
        n310 = Concatenate Strings(w1489, "-stressI-" ("Substring"), w1505, w1467, ".txt" ("Substring")) -> (w1503:string)
        n311 = Fract/Exp String To Number(string=w1502) -> (number=w1477:dbl[])  [unwired: 3 in, 1 out]
        n312 = Index Array(array=w1477, index=1 ("Index")) -> (element=w1473:dbl)
        n313 = Index Array(array=w1477, index=0 ("Index")) -> (element=w1474:dbl)
        n314 = call "4155C Config I Stress.vi"("VISA session"=w1508, "IDG"=w1474, "VDG compliance"=w1473, "error in (no error)"=w1507, "Display on/off"=TRUE) -> ("dup VISA resource name"=w1510:refnum<visa-resource-name>, "error out"=w1509:errorcluster)
        n315 = Index Array(array=w1477, index=2 ("Index")) -> (element=w1475:dbl)
        n316 = String To Path(string=w1503) -> (path=w1493:path)
        n317 = call "4155C Apply Stress.vi"("error in (no error)"=w1509, "Duration"=w1475, "Emergency Stop"=w1488, "VISA resource name in"=w1510) -> ("error out"=w1486:errorcluster, "VISA Resource Name out"=w1484:refnum<visa-resource-name>)
        n318 = VISA Write(VISA resource name=w1484, write buffer=":DISP ON" ("write buffer (\"\")"), error in (no error)=w1486) -> (VISA resource name out=w1483:refnum<visa-resource-name>, error out=w1485:errorcluster)  [unwired: 1 out]
        n319 = call <vilib>:"compatOverwrite.vi"("overwrite (F)"=TRUE) -> ("overwrite?"=w1472:T7)
        n320 = Open/Create/Replace File(file path (use dialog)=w1493, error in=w1485, operation (0:open)=w1472) -> (refnum out=w1496:refnum<file>, error out=w1495:errorcluster)  [unwired: 3 in, 1 out]
        n321 = call "4155C Write array to file.vi"("Byte Stream File Refnum"=w1496, "Header"=string[] ["I stress completed successfully", ""], "error in (no error)"=w1495) -> ("dup refnum"=w1498:refnum<file>, "error out"=w1497:errorcluster)  [unwired: 2 in]
        n322 = Close File(refnum=w1498, error in=w1497) -> (error out=w1491:errorcluster)  [unwired: 1 out]
      }
      frame "vsu2pulse" {
        n323 = Number To Decimal String(number=w1531) -> (decimal integer string=w1566:string)  [unwired: 1 in]
        n324 = Concatenate Strings(w1551, "-vsu2-" ("Substring"), w1566, w1530, ".txt" ("Substring")) -> (w1564:string)
        n325 = Fract/Exp String To Number(string=w1563) -> (number=w1539:dbl[])  [unwired: 3 in, 1 out]
        n326 = String To Path(string=w1564) -> (path=w1555:path)
        n327 = Index Array(array=w1539, index=1 ("Index")) -> (element=w1538:dbl)
        n328 = Index Array(array=w1539, index=0 ("Index")) -> (element=w1536:dbl)
        n329 = call "4155C Config VSU2 Stress.vi"("error in (no error)"=w1568, "VSU2"=w1536, "Display on/off"=TRUE, "VISA session"=w1569) -> ("error out"=w1570:errorcluster, "dup VISA resource name"=w1571:refnum<visa-resource-name>)
        n330 = call "4155C Apply Stress.vi"("error in (no error)"=w1570, "Duration"=w1538, "Emergency Stop"=w1550, "VISA resource name in"=w1571) -> ("error out"=w1548:errorcluster, "VISA Resource Name out"=w1546:refnum<visa-resource-name>)
        n331 = VISA Write(VISA resource name=w1546, write buffer=":DISP ON" ("write buffer (\"\")"), error in (no error)=w1548) -> (VISA resource name out=w1545:refnum<visa-resource-name>, error out=w1547:errorcluster)  [unwired: 1 out]
        n332 = call <vilib>:"compatOverwrite.vi"("overwrite (F)"=TRUE) -> ("overwrite?"=w1535:T7)
        n333 = Open/Create/Replace File(file path (use dialog)=w1555, error in=w1547, operation (0:open)=w1535) -> (refnum out=w1558:refnum<file>, error out=w1557:errorcluster)  [unwired: 3 in, 1 out]
        n334 = call "4155C Write array to file.vi"("Byte Stream File Refnum"=w1558, "Header"=string[] ["VSU2 pulse completed successfully", ""], "error in (no error)"=w1557) -> ("dup refnum"=w1560:refnum<file>, "error out"=w1559:errorcluster)  [unwired: 2 in]
        n335 = Close File(refnum=w1560, error in=w1559) -> (error out=w1553:errorcluster)  [unwired: 1 out]
      }
      frame "sample-fpp" {
        w1603 = string[] ["Time /s", "Id VgVd /A", "Ig VgVd /A", "Vp1 VgVd /V", "Vp2 VgVd /V"] ("Header")
        w1607 = "%d" ("format string")
        n336 = Number To Decimal String(number=w1592) -> (decimal integer string=w1655:string)  [unwired: 1 in]
        n337 = Fract/Exp String To Number(string=w1652) -> (number=w1640:dbl[])  [unwired: 3 in, 1 out]
        n338 = Concatenate Strings(w1646, "-samplefpp-" ("Substring"), w1655, w1591, ".txt" ("Substring")) -> (w1653:string)
        n339 = String To Path(string=w1653) -> (path=w1615:path)
        n340 = Index Array(array=w1640, index=0 ("Index")) -> (element=w1601:dbl)
        n341 = Index Array(array=w1640, index=1 ("Index")) -> (element=w1600:dbl)
        n342 = Index Array(array=w1640, index=2 ("Index")) -> (element=w1648:dbl)
        n343 = Index Array(array=w1640, index=3 ("Index")) -> (element=w1638:dbl)
        n344 = call "4155C Config Sampling Measurements FPP.vi"("VISA session"=w1658, "Num Points"=w1648, "Vg"=w1601, "Display on/off"=TRUE, "Gate Compliance"=w1647, "Drain Compliance"=w1656, "Standby"="Standby", "error in (no error)"=w1657, "Timings"=w1645, "Vd"=w1600, "Sample time"=w1638) -> ("dup VISA resource name"=w1617:refnum<visa-resource-name>, "error out"=w1616:errorcluster)  [unwired: 3 in]
        n345 = Number To Decimal String(number=w1601) -> (decimal integer string=w1627:string)  [unwired: 1 in]
        n346 = call "4155C Take Sample FPP.vi"("VISA resource name in"=w1617, "error in (no error)"=w1616, "Emergency Stop"=w1618) -> ("Time"=w1622:dbl[], "Vp1"=w1632:dbl[], "VISA Resource Name out"=w1598:refnum<visa-resource-name>, "Ig"=w1620:dbl[], "Id"=w1621:dbl[], "Vp2"=w1630:dbl[], "error out"=w1619:errorcluster)  [unwired: 10 in]
        n347 = Insert Into Array(array=dbl[][] [] ("Input Array"), new element=w1622) -> (w1636:dbl[][])  [unwired: 2 in]
        n348 = Number To Decimal String(number=w1600) -> (decimal integer string=w1625:string)  [unwired: 1 in]
        n349 = Insert Into Array(array=w1636, new element=w1621) -> (w1635:dbl[][])  [unwired: 2 in]
        n350 = Concatenate Strings("(Vg = " ("Substring"), w1627, "V, Vd = " ("Substring"), w1625, "V)" ("Substring")) -> (w1623:string)
        n351 = Insert Into Array(array=w1635, new element=w1620) -> (w1634:dbl[][])  [unwired: 2 in]
        n352 = Insert Into Array(array=w1634, new element=w1632) -> (w1631:dbl[][])  [unwired: 2 in]
        n353 = Insert Into Array(array=w1631, new element=w1630) -> (w1599:dbl[][])  [unwired: 2 in]
        n354 = Transpose 2D Array(2D array=w1599) -> (transposed array=w1629:dbl[][])
        n355 = call <vilib>:"compatOverwrite.vi"("overwrite (F)"=TRUE) -> ("overwrite?"=w1596:T7)
        n356 = Open/Create/Replace File(file path (use dialog)=w1615, error in=w1619, operation (0:open)=w1596) -> (refnum out=w1612:refnum<file>, error out=w1613:errorcluster)  [unwired: 3 in, 1 out]
        n357 = Array To Spreadsheet String(array=w1603, 3:w1607) -> (spreadsheet string=w1609:string)  [unwired: 1 in]
        n358 = Search and Replace String(replace all?=TRUE ("replace all? (F)"), input string=w1609, search string="VgVd", replace string=w1623) -> (result string=w1605:string)  [unwired: 4 in, 3 out]
        n359 = Spreadsheet String To Array(format string=w1607, spreadsheet string=w1605, array type (2D Dbl)=w1603) -> (array=w1604:string[])  [unwired: 1 in]
        n360 = call "4155C Write array to file.vi"("Byte Stream File Refnum"=w1612, "Header"=w1604, "Data Array"=w1629, "error in (no error)"=w1613) -> ("dup refnum"=w1610:refnum<file>, "error out"=w1611:errorcluster)  [unwired: 1 in]
        n361 = Close File(refnum=w1610, error in=w1611) -> (error out=w1597:errorcluster)  [unwired: 1 out]
      }
      frame "resample-fpp" {
        w1692 = string[] ["Time /s", "Id VgVd /A", "Ig VgVd /A", "Vp1 VgVd /V", "Vp2 VgVd /V"] ("Header")
        w1696 = "%d" ("format string")
        n362 = Number To Decimal String(number=w1678) -> (decimal integer string=w1736:string)  [unwired: 1 in]
        n363 = Fract/Exp String To Number(string=w1733) -> (number=w1685:dbl[])  [unwired: 3 in, 1 out]
        n364 = Concatenate Strings(w1729, "-resamplefpp-" ("Substring"), w1736, w1679, ".txt" ("Substring")) -> (w1734:string)
        n365 = String To Path(string=w1734) -> (path=w1704:path)
        n366 = Index Array(array=w1685, index=0 ("Index")) -> (element=w1691:dbl)
        n367 = Index Array(array=w1685, index=1 ("Index")) -> (element=w1690:dbl)
        n368 = Number To Decimal String(number=w1691) -> (decimal integer string=w1714:string)  [unwired: 1 in]
        n369 = call "4155C Take Sample FPP.vi"("VISA resource name in"=w1687, "error in (no error)"=w1686, "Emergency Stop"=w1705) -> ("Time"=w1709:dbl[], "Vp1"=w1719:dbl[], "VISA Resource Name out"=w1689:refnum<visa-resource-name>, "Ig"=w1707:dbl[], "Id"=w1708:dbl[], "Vp2"=w1717:dbl[], "error out"=w1706:errorcluster)  [unwired: 10 in]
        n370 = Insert Into Array(array=dbl[][] [] ("Input Array"), new element=w1709) -> (w1723:dbl[][])  [unwired: 2 in]
        n371 = Number To Decimal String(number=w1690) -> (decimal integer string=w1712:string)  [unwired: 1 in]
        n372 = Insert Into Array(array=w1723, new element=w1708) -> (w1722:dbl[][])  [unwired: 2 in]
        n373 = Concatenate Strings("(Vg = " ("Substring"), w1714, "V, Vd = " ("Substring"), w1712, "V)" ("Substring")) -> (w1710:string)
        n374 = Insert Into Array(array=w1722, new element=w1707) -> (w1721:dbl[][])  [unwired: 2 in]
        n375 = Insert Into Array(array=w1721, new element=w1719) -> (w1718:dbl[][])  [unwired: 2 in]
        n376 = Insert Into Array(array=w1718, new element=w1717) -> (w1684:dbl[][])  [unwired: 2 in]
        n377 = call <vilib>:"compatOverwrite.vi"("overwrite (F)"=TRUE) -> ("overwrite?"=w1683:T7)
        n378 = Open/Create/Replace File(file path (use dialog)=w1704, error in=w1706, operation (0:open)=w1683) -> (refnum out=w1701:refnum<file>, error out=w1702:errorcluster)  [unwired: 3 in, 1 out]
        n379 = Array To Spreadsheet String(array=w1692, 3:w1696) -> (spreadsheet string=w1698:string)  [unwired: 1 in]
        n380 = Transpose 2D Array(2D array=w1684) -> (transposed array=w1716:dbl[][])
        n381 = Search and Replace String(replace all?=TRUE ("replace all? (F)"), input string=w1698, search string="VgVd", replace string=w1710) -> (result string=w1694:string)  [unwired: 4 in, 3 out]
        n382 = Spreadsheet String To Array(format string=w1696, spreadsheet string=w1694, array type (2D Dbl)=w1692) -> (array=w1693:string[])  [unwired: 1 in]
        n383 = call "4155C Write array to file.vi"("Byte Stream File Refnum"=w1701, "Header"=w1693, "Data Array"=w1716, "error in (no error)"=w1702) -> ("dup refnum"=w1699:refnum<file>, "error out"=w1700:errorcluster)  [unwired: 1 in]
        n384 = Close File(refnum=w1699, error in=w1700) -> (error out=w1688:errorcluster)  [unwired: 1 out]
      }
      frame "serial" {
        n385 = local read "Termination char\n(0xA = '\\n' = LF)\n(0xD = '\\r' = CR)"() -> (w1764:u8)
        n386 = local read "Enable Termination\nChar (T)"() -> (w1765:bool)
        n387 = Index Array(array=w1772, index=0 ("Index")) -> (element=w1771:string)
        n388 = local read "parity"() -> (w1755:u16)
        n389 = local read "Delay before read (ms)"() -> (w1766:u32)
        n390 = local read "byte count"() -> (w1763:u32)
        n391 = local read "Timeout (ms)"() -> (w1762:u32)
        n392 = local read "VISA resource name"() -> (w1759:refnum<visa-resource-name>)
        n393 = local read "baud rate"() -> (w1758:u32)
        n394 = local read "Serial End Mode for Reads"() -> (w1757:u16)
        n395 = local read "data bits"() -> (w1756:u16)
        n396 = local read "stop bits"() -> (w1761:u16)
        n397 = local read "flow control"() -> (w1760:u16)
        n398 = call "Serial write and read v0.5.vi"("Delay before read (ms)"=w1766, "Termination char\n(0xA = '\\n' = LF)\n(0xD = '\\r' = CR)"=w1764, "Enable Termination\nChar (T)"=w1765, "parity"=w1755, "stop bits"=w1761, "string to write"=w1771, "flow control"=w1760, "byte count"=w1763, "Serial Settings:Serial End Mode for Reads"=w1757, "Timeout (ms)"=w1762, "error in (no error)"=w1777, "VISA resource name"=w1759, "baud rate"=w1758, "data bits"=w1756) -> ("read string"=w1767:string, "error out"=w1776:errorcluster)
        n399 = Build Array (concatenate)(w1767, w1768) -> (w1769:string[])
      }
      frame "pump" {
        # "Time array for valve position"
        # "Time array for absolute plunger position"
        # "Valve position"
        # "Absolute plunger position"
        # "Remove \"_\""
        # "Check if hard stop is pressed."
        # "Check if halt is pressed."
        # "Check if pump is idle. Else halt."
        n400 = Index Array(array=w1842, index=0 ("Index")) -> (element=w1819:string)
        n401 = case shown="\"No error\", Default" w1817 {
          tunnel: w1819 -> [w1878 _ w1880 w1881 w1882 w1883 _ _ w1886 w1887 _]
          tunnel: [w1878 "/1H" w1880 w1881 w1882 w1883 "/1H" "/1H" w1886 w1887 "/1H"] -> w1818
          frame "No error", Default {
          }
          frame "Initialization" {
          }
          frame "Invalid command" {
          }
          frame "Invalid operand" {
          }
          frame "Device not initialized" {
          }
          frame "Internal failure" {
          }
          frame "Plunger overload" {
          }
          frame "Valve overload" {
          }
          frame "Plunger move not allowed" {
          }
          frame "A/D converter failure" {
          }
          frame "Command overflow" {
          }
        }
        n402 = local read "Hard stop pump"() -> (w1821:bool)
        n403 = local read "Halt pump"() -> (w1824:bool)
        n404 = local read "Serial End Mode for Reads"() -> (w1830:u16)
        n405 = local read "flow control"() -> (w1833:u16)
        n406 = local read "stop bits"() -> (w1834:u16)
        n407 = local read "parity"() -> (w1828:u16)
        n408 = local read "Delay before read (ms)"() -> (w1839:u32)
        n409 = local read "byte count"() -> (w1836:u32)
        n410 = local read "Timeout (ms)"() -> (w1835:u32)
        n411 = local read "VISA resource name"() -> (w1832:refnum<visa-resource-name>)
        n412 = local read "baud rate"() -> (w1831:u32)
        n413 = local read "Enable Termination\nChar (T)"() -> (w1838:bool)
        n414 = local read "Termination char\n(0xA = '\\n' = LF)\n(0xD = '\\r' = CR)"() -> (w1837:u8)
        n415 = case shown="True" w1824 {
          tunnel: [w1892 "/1H"] -> w1823
          tunnel: w1818 -> [w1892 _]
          frame False {
          }
          frame True {
            n416 = local write "Halt pump"(FALSE) -> ()
          }
        }
        n417 = case shown="True" w1821 {
          tunnel: [w1889 "/1T"] -> w1822
          tunnel: w1823 -> [w1889 _]
          frame False {
          }
          frame True {
            n418 = local write "Hard stop pump"(FALSE) -> ()
          }
        }
        n419 = local read "data bits"() -> (w1829:u16)
        n420 = String Subset(string=w1813, offset (0)=1) -> (substring=w1811:string)  [unwired: 1 in]
        n421 = call "SPM Pump v0.6.vi"("Termination char\n(0xA = '\\n' = LF)\n(0xD = '\\r' = CR)"=w1837, "Enable Termination\nChar (T)"=w1838, "Timeout (ms)"=w1835, "Serial Settings:Serial End Mode for Reads"=w1830, "byte count"=w1836, "Delay before read (ms)"=w1839, "Time <input>"=w1816, "error in (no error)"=w1847, "Serial port input"=w1822, "VISA resource name"=w1832, "parity"=w1828, "baud rate"=w1831, "stop bits"=w1834, "data bits"=w1829, "flow control"=w1833, "Time units <input>"=w1811) -> ("Input command"=w1810:string, "Serial port data"=w1800:string[], "Pump status"=w1806:string, "Valve position"=w1808:i32, "Absolute plunger position"=w1820:i32, "Serial port"=w1815:string, "error out"=w1846:errorcluster)  [unwired: 1 in, 4 out]
        n422 = case shown="\"?6\"" w1810 {
          tunnel: [w1859 w1867 w1873] -> w1827
          tunnel: w1826 -> [w1859 w1866 w1873]
          tunnel: w1820 -> [_ w1865 _]
          tunnel: w1807 -> [w1858 w1864 w1874]
          tunnel: [w1858 w1864 w1876] -> w1809
          tunnel: w1808 -> [_ _ w1875]
          tunnel: w1805 -> [_ w1863 w1871]
          tunnel: w1804 -> [w1857 w1862 w1872]
          tunnel: [w1857 w1861 w1872] -> w1803
          tunnel: [w1856 w1860 w1870] -> w1802
          tunnel: w1801 -> [w1856 w1860 w1869]
          frame "Q", Default {
          }
          frame "?" {
            n423 = Build Array (concatenate)(w1866, w1865) -> (w1867:i32[])
            n424 = Build Array (concatenate)(w1862, w1863) -> (w1861:i32[])
            n425 = call "4155C Split array.vi"("X data in"=w1861, "Y1 data in"=w1867) -> ("Array of clusters"=w1868:cluster{"Y data in":dbl[], "X data in":dbl[]}[])  [unwired: 5 in, 1 out]
            n426 = local write "Absolute plunger position vs time"(w1868) -> ()
          }
          frame "?6" {
            n427 = Build Array (concatenate)(w1874, w1875) -> (w1876:i32[])
            n428 = Build Array (concatenate)(w1869, w1871) -> (w1870:i32[])
            n429 = call "4155C Split array.vi"("X data in"=w1870, "Y1 data in"=w1876) -> ("Array of clusters"=w1877:cluster{"Y data in":dbl[], "X data in":dbl[]}[])  [unwired: 5 in, 1 out]
            n430 = local write "Valve position vs time"(w1877) -> ()
          }
        }
        n431 = Build Array (concatenate)(w1798, w1800) -> (w1799:string[][])
        n432 = Build Array (concatenate)(w1814, w1815) -> (w1840:string[])
      }
      frame "filename" {
        n433 = Index Array(array=w1896, index=0 ("Index")) -> (element=w1895:string)
      }
    }
    n434 = Build Array(w137, w66, w76, w75, w74, w73, w72, w71, w70, w69, w68, w67, w65) -> (w176:dbl[][])
    n435 = Transpose 2D Array(2D array=w176) -> (transposed array=w175:dbl[][])
    n436 = Concatenate Strings(w117, w60, "Imax_Imin_Ion_Ioff_vs_time.txt" ("Suffix (Imax,Imin,Ion,Ioff)")) -> (w186:string)
    n437 = Build Array(w98, "Is max (A)" ("VAR2 Name"), "Is min (A)" ("VAR2 Name"), "Id max (A)" ("VAR2 Name"), "Id min (A)" ("VAR2 Name"), "Ig max (A)" ("VAR2 Name"), "Ig min (A)" ("VAR2 Name"), "Is on (A)" ("VAR2 Name"), "Is off (A)" ("VAR2 Name"), "Id on (A)" ("VAR2 Name"), "Id off (A)" ("VAR2 Name"), "Ig on (A)" ("VAR2 Name"), "Ig off (A)" ("VAR2 Name")) -> (w181:string[])
    n438 = Array To Spreadsheet String(array=w175, 3:"%e" ("format string")) -> (spreadsheet string=w179:string)  [unwired: 1 in]
    n439 = Array To Spreadsheet String(array=w181, 3:"" ("format string")) -> (spreadsheet string=w180:string)  [unwired: 1 in]
    n440 = String To Path(string=w186) -> (path=w185:path)
    n441 = Build Array(w180, w179) -> (w178:string[])
    n442 = Write to Text File(file (use dialog)=w185, text=w178, error in=w133) -> (refnum out=w187:refnum<file>, error out=w177:errorcluster)  [unwired: 1 in, 1 out]
    n443 = Close File(refnum=w187, error in=w177) -> (error out=w116:errorcluster)  [unwired: 1 out]
    n444 = Build Array(w112, w138) -> (w143:i32[][])
    n445 = Build Array(w98, "Absolute plunger position" ("VAR2 Name")) -> (w146:string[])
    n446 = Transpose 2D Array(2D array=w143) -> (transposed array=w136:i32[][])
    n447 = Array To Spreadsheet String(array=w146, 3:"" ("format string")) -> (spreadsheet string=w145:string)  [unwired: 1 in]
    n448 = Array To Spreadsheet String(array=w136, 3:"%e" ("format string")) -> (spreadsheet string=w142:string)  [unwired: 1 in]
    n449 = Build Array(w145, w142) -> (w148:string[])
    n450 = Concatenate Strings(w117, w60, "plunger_vs_time.txt" ("Suffix (plunger)")) -> (w140:string)
    n451 = String To Path(string=w140) -> (path=w139:path)
    n452 = Write to Text File(file (use dialog)=w139, text=w148, error in=w116) -> (refnum out=w141:refnum<file>, error out=w150:errorcluster)  [unwired: 1 in, 1 out]
    n453 = Close File(refnum=w141, error in=w150) -> (error out=w115:errorcluster)  [unwired: 1 out]
    n454 = Concatenate Strings(w117, w60, "serial_port_output.txt" ("Suffix (serial port log)")) -> (w156:string)
    n455 = String To Path(string=w156) -> (path=w155:path)
    n456 = Build Array(w98, "Serial port input" ("VAR2 Name"), "Pump status" ("VAR2 Name"), "Serial port output: ") -> (w102:string[])
    n457 = Array To Spreadsheet String(array=w108, 3:"" ("format string")) -> (spreadsheet string=w99:string)  [unwired: 1 in]
    n458 = Array To Spreadsheet String(array=w102, 3:"" ("format string")) -> (spreadsheet string=w100:string)  [unwired: 1 in]
    n459 = Build Array(w100, w99) -> (w101:string[])
    n460 = Array To Spreadsheet String(array=w107, 3:"" ("format string")) -> (spreadsheet string=w161:string)  [unwired: 1 in]
    n461 = Write to Text File(file (use dialog)=w155, text=w101, error in=w115) -> (refnum out=w157:refnum<file>, error out=w158:errorcluster)  [unwired: 1 in, 1 out]
    n462 = Close File(refnum=w157, error in=w158) -> (error out=w114:errorcluster)  [unwired: 1 out]
    n463 = local write "Serial port data"(w161) -> ()
    n464 = Build Array(w111, w119) -> (w125:i32[][])
    n465 = Build Array(w98, "Valve port" ("VAR2 Name")) -> (w128:string[])
    n466 = Transpose 2D Array(2D array=w125) -> (transposed array=w120:i32[][])
    n467 = Array To Spreadsheet String(array=w128, 3:"" ("format string")) -> (spreadsheet string=w127:string)  [unwired: 1 in]
    n468 = Array To Spreadsheet String(array=w120, 3:"%e" ("format string")) -> (spreadsheet string=w124:string)  [unwired: 1 in]
    n469 = Build Array(w127, w124) -> (w130:string[])
    n470 = Concatenate Strings(w117, w60, "valve_port_vs_time.txt" ("Suffix (valve)")) -> (w122:string)
    n471 = String To Path(string=w122) -> (path=w121:path)
    n472 = Write to Text File(file (use dialog)=w121, text=w130, error in=w114) -> (refnum out=w123:refnum<file>, error out=w132:errorcluster)  [unwired: 1 in, 1 out]
    n473 = Close File(refnum=w123, error in=w132) -> (error out=w113:errorcluster)  [unwired: 1 out]
  }
  "error out" <- w18
